vi "数据表比对.vi"(8 "error in (no error)":errorcluster, 9 "查询元素输入":string(combo), 10 "仪器日志参数":string, 11 "table输入":string(combo)) -> (0 "error out":errorcluster, 1 "columns输出":string[](array[string]), 2 "待发送第一条数据":string[](array[string]), 3 "待发送数据":string[][](table))   [LabVIEW 2016, in "数据传输系统-03.lvlib"]
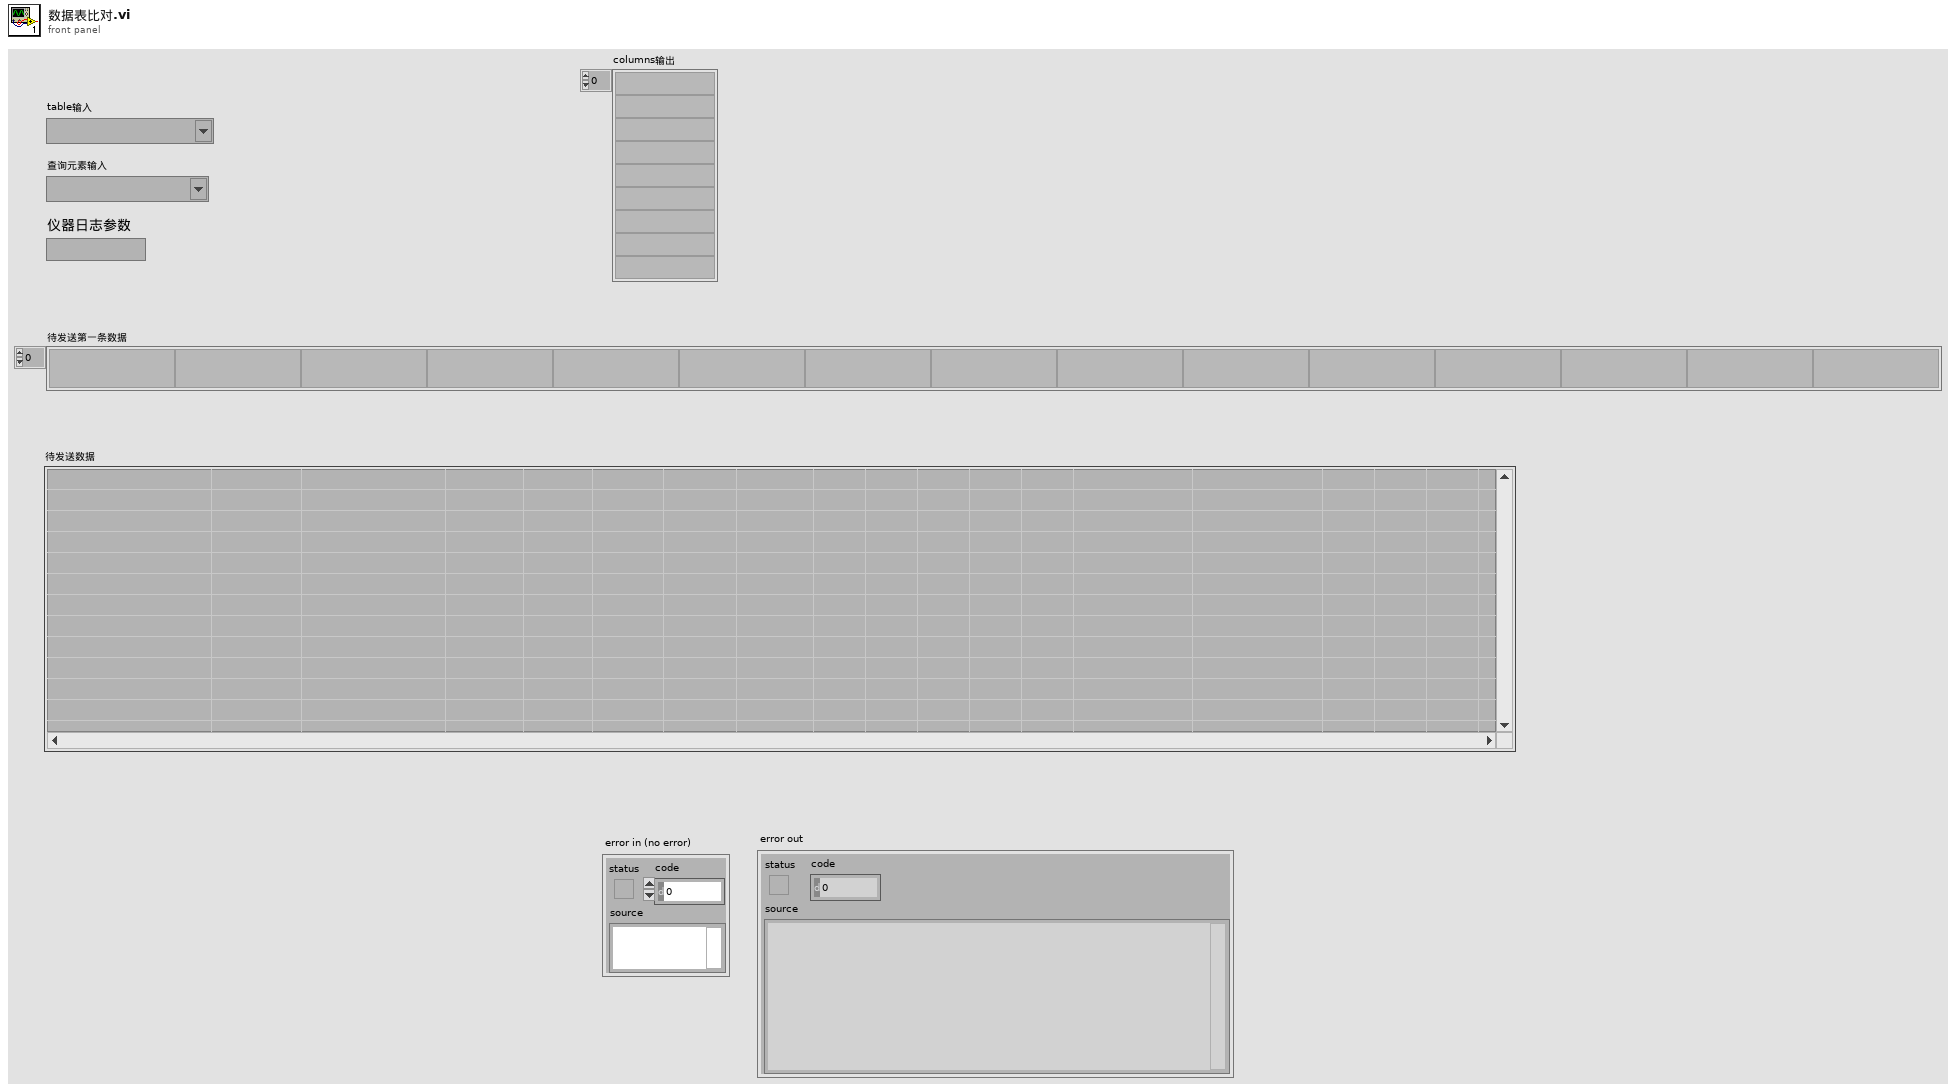
[diagram p1: front panel]
types:
  T1 = cluster{"氨氮仪器日志索引起始时间":string, "总磷仪器日志索引起始时间":string, "总氮仪器日志索引起始时间":string, "CODMn仪器日志索引起始时间":string, "CODCr仪器日志索引起始时间":string, "系统仪器日志索引起始时间":string, "氟化物仪器日志索引起始时间":string}
  T2 = cluster{"氨氮仪器参数索引起始时间":string, "总磷仪器参数索引起始时间":string, "总氮仪器参数索引起始时间":string, "CODMn仪器参数索引起始时间":string, "CODCr仪器参数索引起始时间":string, "DO仪器参数索引起始时间":string, "PH仪器参数索引起始时间":string, "比电导率仪器参数索引起始时间":string, "水温仪器参数索引起始时间":string, "浊度仪器参数索引起始时间":string, "叶绿素a仪器参数索引起始时间":string, "藻密度仪器参数索引起始时间":string, "ORP仪器参数索引起始时间":string, "氟化物仪器参数索引起始时间":string}
  T3 = cluster{"氨氮报警信息索引起始时间":string, "总磷报警信息索引起始时间":string, "总氮报警信息索引起始时间":string, "CODMn报警信息索引起始时间":string, "CODCr报警信息索引起始时间":string, "DO报警信息索引起始时间":string, "PH报警信息索引起始时间":string, "比电导率报警信息索引起始时间":string, "水温报警信息索引起始时间":string, "浊度报警信息索引起始时间":string, "叶绿素报警信息索引起始时间":string, "系统报警信息索引起始时间":string, "氟化物报警信息索引起始时间":string}
  T4 = cluster{"氨氮零点核查索引起始时间":string, "总磷零点核查索引起始时间":string, "总氮零点核查索引起始时间":string, "CODMn零点核查索引起始时间":string, "CODCr零点核查索引起始时间":string, "亚硝酸盐零点核查索引起始时间":string, "硫化物零点核查索引起始时间":string, "ORP零点核查索引起始时间":string, "氟化物零点核查索引起始时间":string}
  T5 = cluster{"氨氮标样核查索引起始时间":string, "总磷标样核查索引起始时间":string, "总氮标样核查索引起始时间":string, "CODMn标样核查索引起始时间":string, "CODCr标样核查索引起始时间":string, "DO标样核查索引起始时间":string, "PH标样核查索引起始时间":string, "比电导率标样核查索引起始时间":string, "水温标样核查索引起始时间":string, "浊度标样核查索引起始时间":string, "叶绿素a标样核查索引起始时间":string, "藻密度标样核查索引起始时间":string, "亚硝酸盐标样核查索引起始时间":string, "硫化物标样核查索引起始时间":string, "ORP标样核查索引起始时间":string, "氟化物标样核查索引起始时间":string}
  T6 = cluster{"氨氮跨度核查索引起始时间":string, "总磷跨度核查索引起始时间":string, "总氮跨度核查索引起始时间":string, "CODMn跨度核查索引起始时间":string, "CODCr跨度核查索引起始时间":string, "亚硝酸盐跨度核查索引起始时间":string, "硫化物跨度核查索引起始时间":string, "ORP跨度核查索引起始时间":string, "氟化物跨度核查索引起始时间":string}
  T7 = typedef "LVDateTimeRec.ctl" = cluster{"秒数的小数部分":dbl, "秒":i32, "分":i32, "时":i32, "日":i32, "月":i32, "年":i32, "天数（周）":i32, "天数（年）":i32, "DST":i32}
  T8 = cluster{"氨氮加标回收索引起始时间":string, "总磷加标回收索引起始时间":string, "总氮加标回收索引起始时间":string, "CODMn加标回收索引起始时间":string, "CODCr加标回收索引起始时间":string, "氟化物加标回收索引起始时间":string}
  T9 = cluster{"氨氮平行样索引起始时间":string, "总磷平行样索引起始时间":string, "总氮平行样索引起始时间":string, "CODMn平行样索引起始时间":string, "CODCr平行样索引起始时间":string, "氟化物平行样索引起始时间":string}
  T10 = cluster{"氨氮集成干预索引起始时间":string, "总磷集成干预索引起始时间":string, "总氮集成干预索引起始时间":string, "CODMn集成干预索引起始时间":string, "CODCr集成干预索引起始时间":string, "DO集成干预索引起始时间":string, "PH集成干预索引起始时间":string, "比电导率集成干预索引起始时间":string, "水温集成干预索引起始时间":string, "浊度集成干预索引起始时间":string, "叶绿素a集成干预索引起始时间":string, "藻密度集成干预索引起始时间":string, "亚硝酸盐集成干预索引起始时间":string, "硫化物集成干预索引起始时间":string, "ORP集成干预索引起始时间":string, "氟化物集成干预索引起始时间":string}
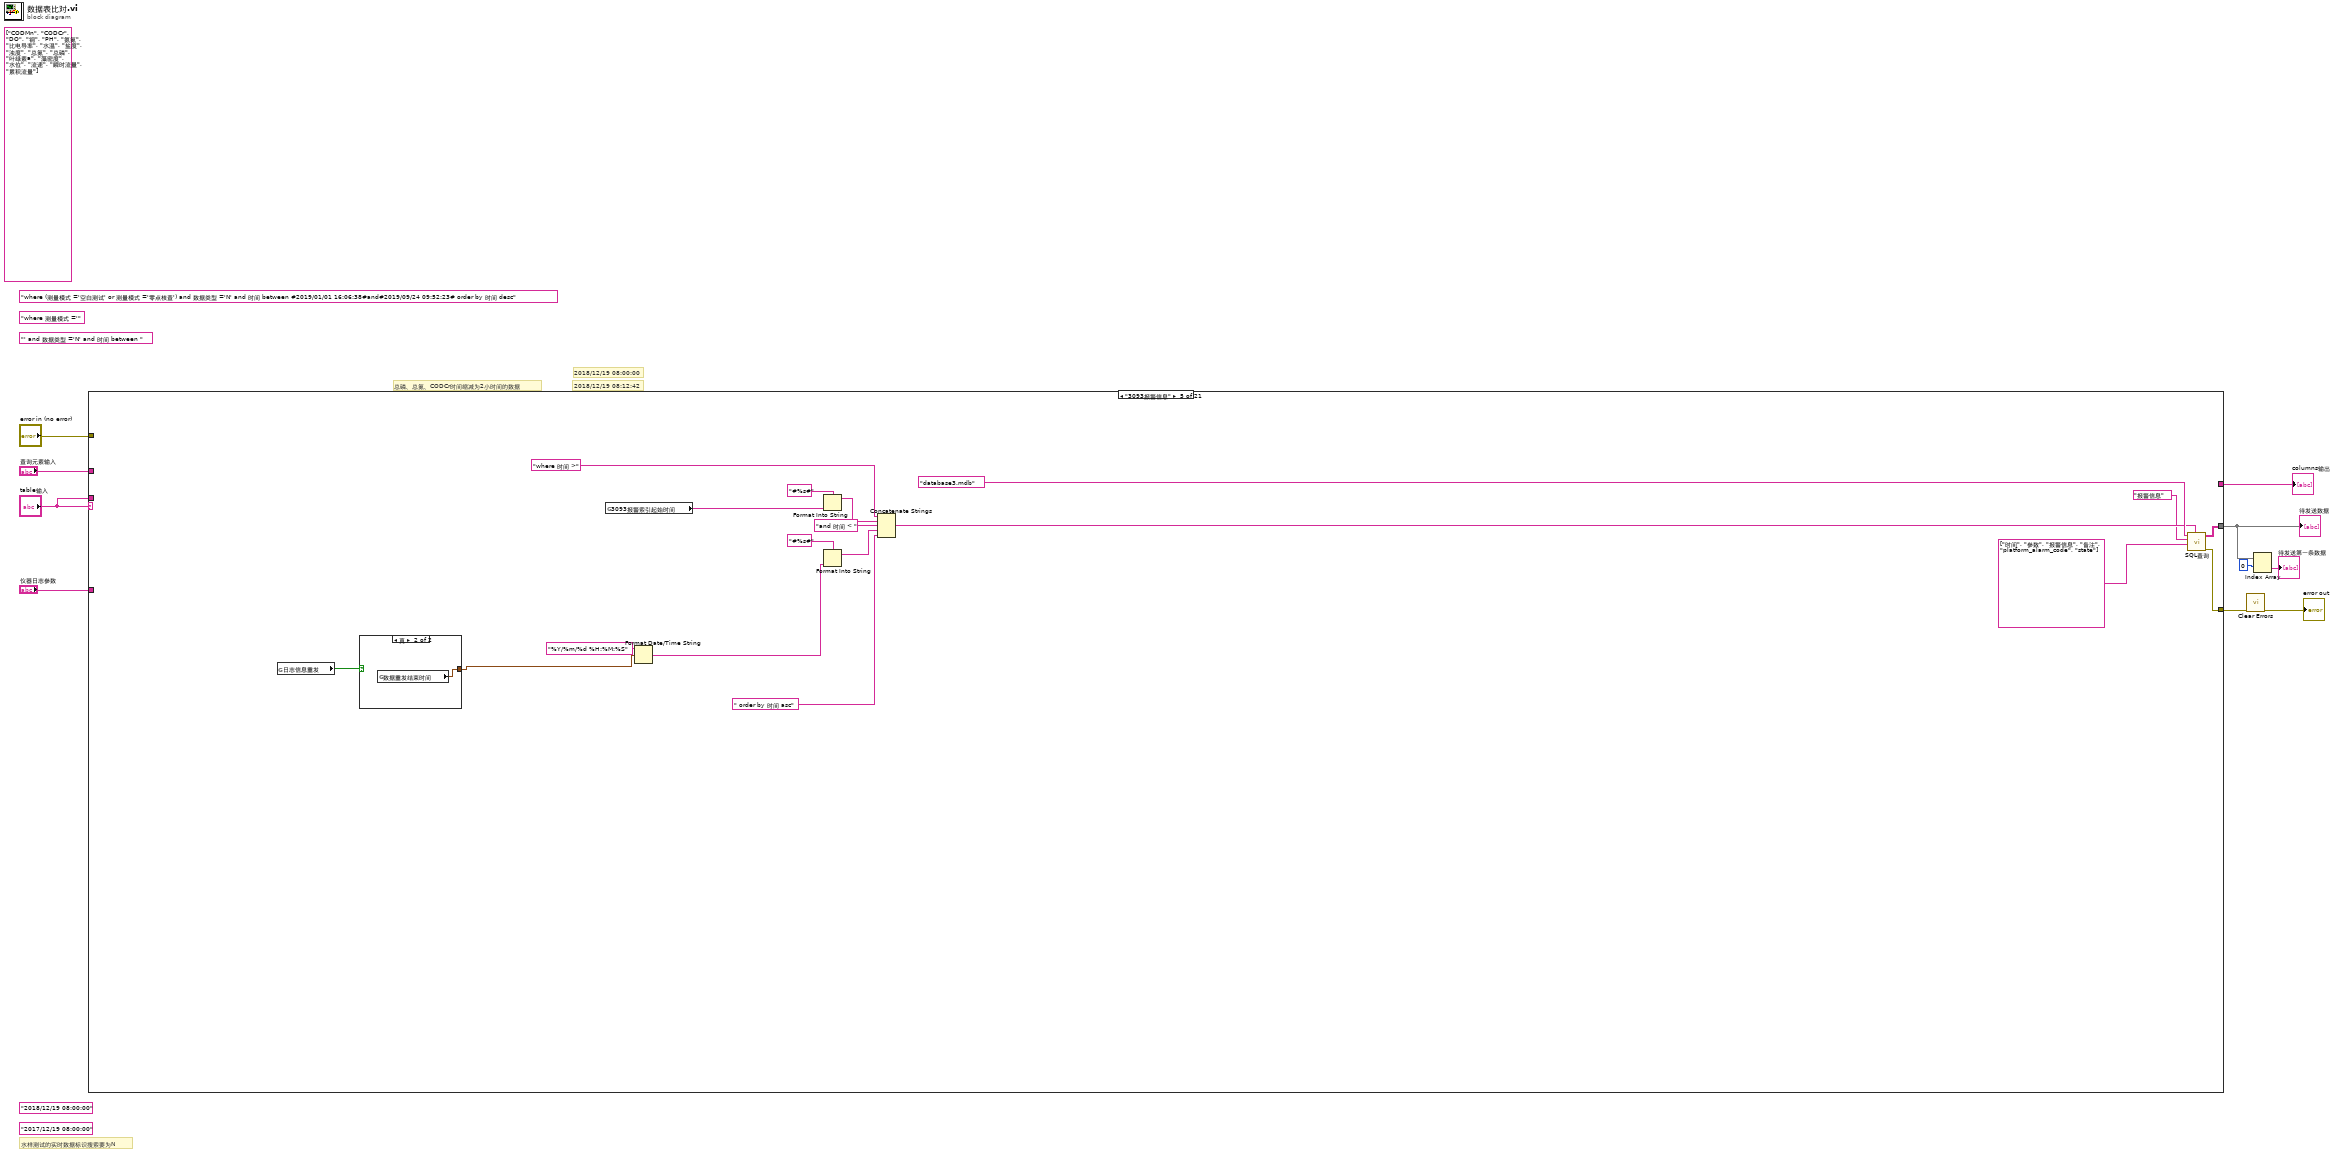
[diagram p0: block diagram]
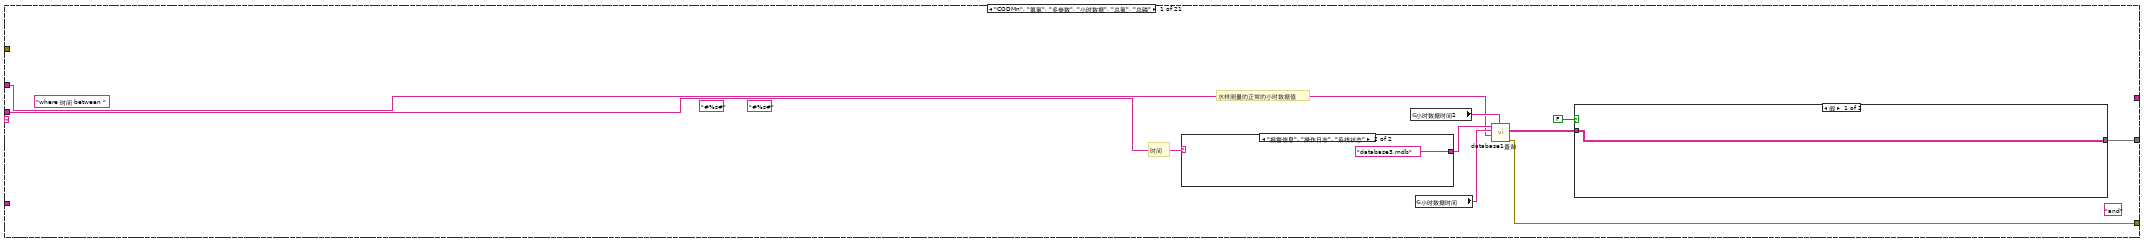
[diagram p2: hidden frame]
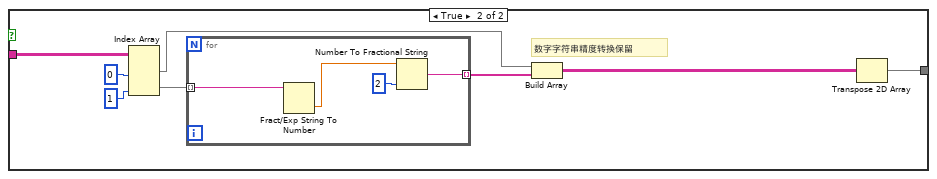
[diagram p3: hidden frame]
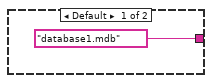
[diagram p4: hidden frame]
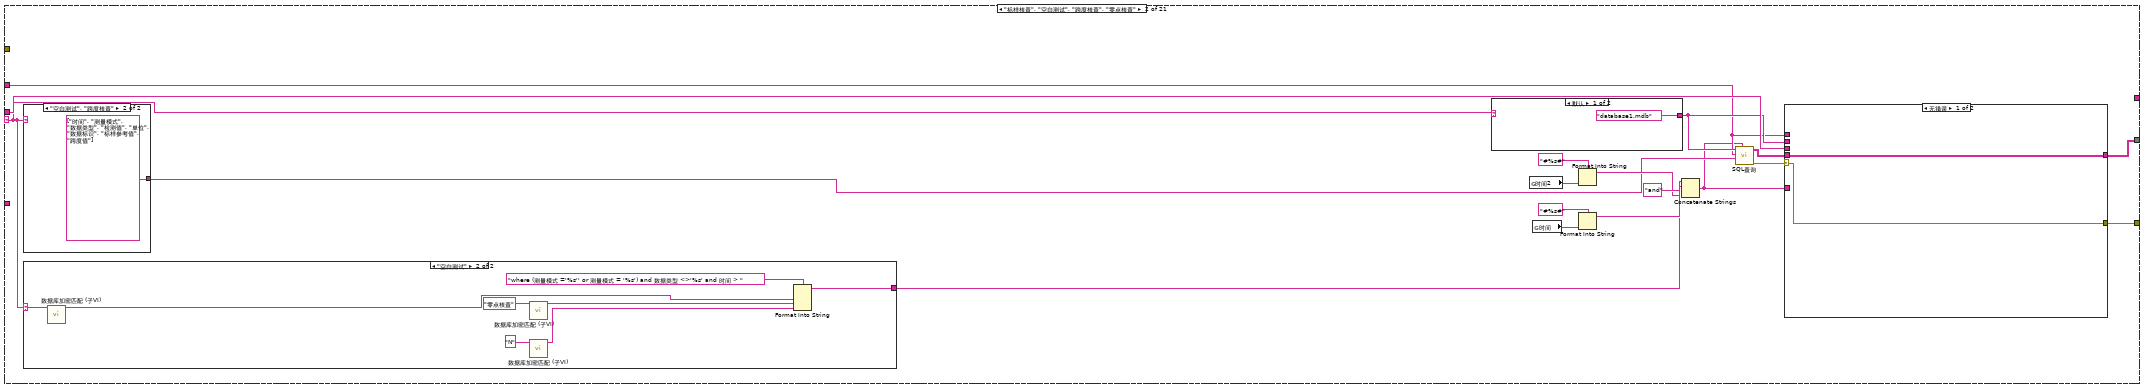
[diagram p5: hidden frame]
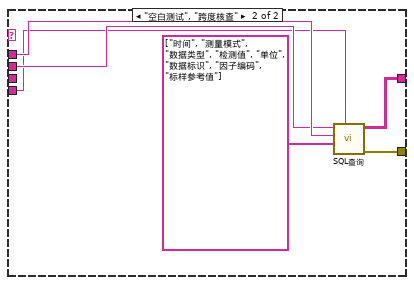
[diagram p7: hidden frame]
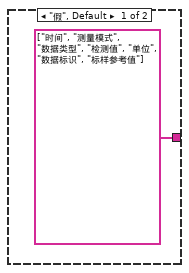
[diagram p8: hidden frame]
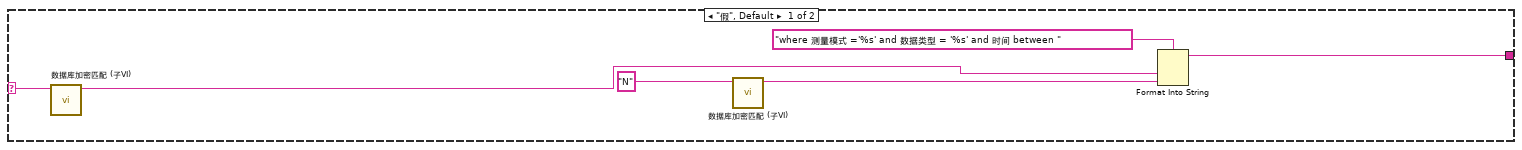
[diagram p9: hidden frame]
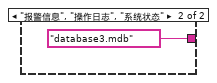
[diagram p10: hidden frame]
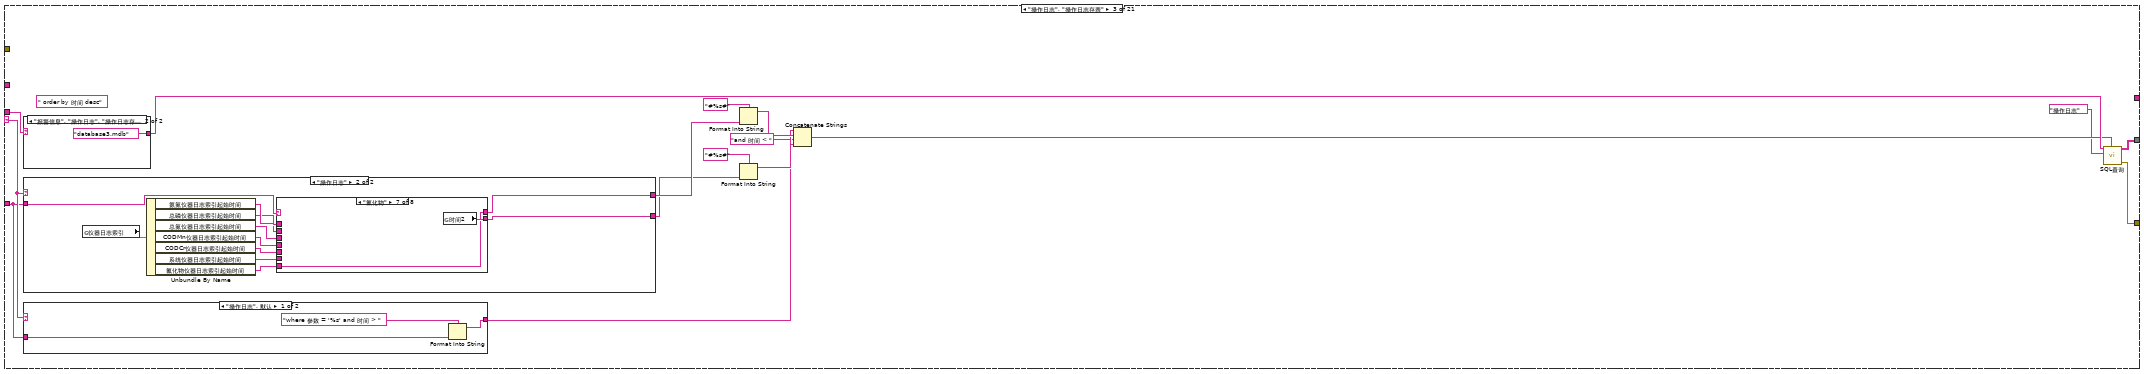
[diagram p11: hidden frame]
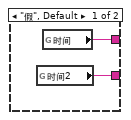
[diagram p12: hidden frame]
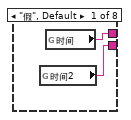
[diagram p13: hidden frame]
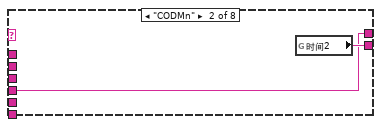
[diagram p14: hidden frame]
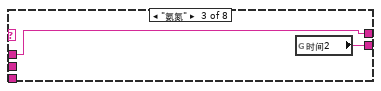
[diagram p15: hidden frame]
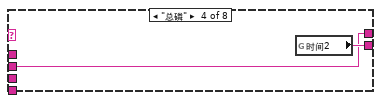
[diagram p16: hidden frame]
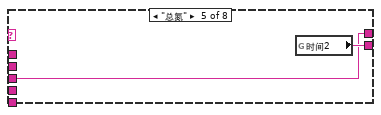
[diagram p17: hidden frame]
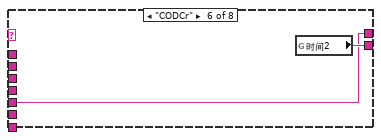
[diagram p18: hidden frame]
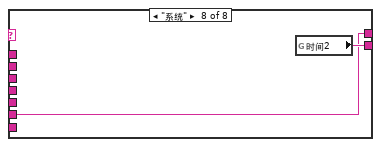
[diagram p19: hidden frame]
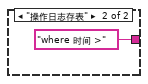
[diagram p20: hidden frame]
diagram:
  (unwired) "' and 数据类型 ='N' and 时间 between "
  (unwired) "where 测量模式 ='" ("condition")
  (unwired) "where (测量模式 ='空白测试' or 测量模式 ='零点核查') and 数据类型 ='N' and 时间 between #2019/01/01 16:06:38#and#2019/09/24 09:52:23# order by 时间 desc" ("condition")
  (unwired) string[] ["CODMn", "CODCr", "DO", "铜", "PH", "氨氮", "比电导率", "水温", "盐度", "浊度", "总氮", "总磷", "叶绿素a", "藻密度", "水位", "流速", "瞬时流量", "累积流量"] ("查询参数数组")
  (unwired) "2017/12/19 08:00:00"
  (unwired) "2018/12/19 08:00:00"
  # "水样测试的实时数据标识搜索要为N"
  # "2018/12/19 08:00:00"
  # "总磷、总氮、CODCr时间缩减为2小时间的数据"
  # "2018/12/19 08:12:42"
  n1 = case shown="\"3093报警信息\"" "table输入" {
    selector: "table输入" -> [_ w41 w91 _ _ _ _ _ _ w389 _ _ _ _ _ _ _ _ _ _ _]
    tunnel: "error in (no error)" -> [_ _ _ _ _ _ _ _ _ _ _ _ w500 _ _ _ _ _ _ _ _]
    tunnel: [w17 w35 w100 w153 w173 w192 w201 w260 w364 w403 w489 w497 w500 w501 w686 w731 w796 w865 w907 w950 w1001] -> w8
    tunnel: [w13 w36 w98 w151 w171 w190 w228 w262 w356 w401 w469 w496 w498 w503 w684 w734 w794 w868 w910 w953 w1003] -> w1
    tunnel: "table输入" -> [w19 w52 w102 _ _ _ w200 w263 _ w393 _ w493 _ _ _ _ _ _ _ _ _]
    tunnel: "查询元素输入" -> [w11 w39 _ _ _ _ _ _ _ _ _ _ _ w507 w671 w716 w782 w857 w899 w940 w997]
    tunnel: "仪器日志参数" -> [_ _ w88 _ _ w178 w195 w251 w335 w388 w468 _ _ _ _ _ _ _ _ _ _]
    tunnel: [_ _ _ _ _ _ _ _ _ _ _ w492 _ _ _ _ _ _ _ _ _] -> w2
    frame "CODMn", "氨氮", "多参数", "小时数据", "总氮", "总磷" {
      (unwired) "and" ("字符串")
      (unwired) "#%s#" ("初始字符串")
      (unwired) "#%s#" ("初始字符串")
      (unwired) "where 时间 between " ("condition")
      # "水样测量的正常的小时数据值"
      # "时间"
      n2 = case shown="\"报警信息\", \"操作日志\", \"系统状态\"" w19 {
        tunnel: ["database1.mdb" ("database") "database3.mdb" ("database")] -> w18
        frame Default {
        }
        frame "报警信息", "操作日志", "系统状态" {
        }
      }
      n3 = global read "全局 时间2.vi" "小时数据时间2"() -> (w15:string)
      n4 = global read "全局 水样时间.vi" "小时数据时间"() -> (w16:string)
      n5 = call "database1查询.vi"("时间2"=w15, "table"=w11, "时间1"=w16, "database"=w18) -> ("error out"=w17:errorcluster, "data"=w14:string[][])  [unwired: 4 in, 1 out]
      n6 = case shown="假" FALSE {
        tunnel: w14 -> [w20 w28]
        tunnel: [w20 w21] -> w13
        frame False {
        }
        frame True {
          # "数字字符串精度转换保留"
          n7 = Index Array(array=w28, index (col) #1=0 ("禁用的索引 (列)"), index (col) #2=1 ("索引 (列)")) -> (element #1=w24:string[], element #2=w25:string[])  [unwired: 2 in]
          n8 = for {
            tunnel: w25 -> [w30] mode=indexing
            tunnel: [w29] -> w23 mode=indexing
            n9 = Fract/Exp String To Number(string=w30) -> (number=w31:dbl)  [unwired: 3 in, 1 out]
            n10 = Number To Fractional String(number=w31, precision (6)=i16 2 ("精度(6)")) -> (F-format string=w29:string)  [unwired: 2 in]
          }
          n11 = Build Array(w24, w23) -> (w22:string[][])
          n12 = Transpose 2D Array(2D array=w22) -> (transposed array=w21:string[][])
        }
      }
    }
    frame "标样核查", "空白测试", "跨度核查", "零点核查" {
      n13 = case shown="\"空白测试\", \"跨度核查\"" w41 {
        tunnel: [string[] ["时间", "测量模式", "数据类型", "检测值", "单位", "数据标识", "标样参考值"] ("columns") string[] ["时间", "测量模式", "数据类型", "检测值", "单位", "数据标识", "标样参考值", "跨度值"] ("columns")] -> w43
        frame "假", Default {
        }
        frame "空白测试", "跨度核查" {
        }
      }
      n14 = case shown="\"空白测试\"" w41 {
        selector: w41 -> [w74 w81]
        tunnel: [w75 w83] -> w44
        frame "假", Default {
          n15 = call "数据库加密匹配 (子VI).vi"("输入参数"=w74) -> ("Encoded String"=w73:string)  [unwired: 10 in]
          n16 = call "数据库加密匹配 (子VI).vi"("输入参数"="N" ("字符串")) -> ("Encoded String"=w71:string)  [unwired: 10 in]
          n17 = Format Into String(format string="where 测量模式 ='%s' and 数据类型 = '%s' and 时间 between " ("格式字符串"), w73, w71) -> (resulting string=w75:string)  [unwired: 2 in, 1 out]
        }
        frame "空白测试" {
          n18 = call "数据库加密匹配 (子VI).vi"("输入参数"=w81) -> ("Encoded String"=w82:string)  [unwired: 10 in]
          n19 = call "数据库加密匹配 (子VI).vi"("输入参数"="零点核查") -> ("Encoded String"=w79:string)  [unwired: 10 in]
          n20 = call "数据库加密匹配 (子VI).vi"("输入参数"="N") -> ("Encoded String"=w77:string)  [unwired: 10 in]
          n21 = Format Into String(format string="where (测量模式 ='%s'' or 测量模式 = '%s') and 数据类型 <>'%s' and 时间 > " ("格式字符串"), w82, w79, w77) -> (resulting string=w83:string)  [unwired: 2 in, 1 out]
        }
      }
      n22 = case shown="默认" w52 {
        tunnel: ["database1.mdb" ("database") "database3.mdb" ("database")] -> w40
        frame Default {
        }
        frame "报警信息", "操作日志", "系统状态" {
        }
      }
      n23 = global read "全局 时间2.vi" "时间2"() -> (w45:string)
      n24 = global read "全局 水样时间.vi" "时间"() -> (w46:string)
      n25 = Format Into String(format string="#%s#" ("初始字符串"), w45) -> (resulting string=w47:string)  [unwired: 2 in, 1 out]
      n26 = Format Into String(format string="#%s#" ("初始字符串"), w46) -> (resulting string=w51:string)  [unwired: 2 in, 1 out]
      n27 = Concatenate Strings(w44, w51, "and" ("字符串"), w47) -> (w38:string)
      n28 = call "SQL查询.vi"("condition"=w38, "columns"=w43, "table输入"=w39, "database"=w40) -> ("error out"=w42:errorcluster, "data"=w37:string[][])  [unwired: 4 in, 2 out]
      n29 = case shown="无错误" w42 {
        selector: w42 -> [w53 _]
        tunnel: w41 -> [_ w61]
        tunnel: w39 -> [_ w60]
        tunnel: w40 -> [_ w59]
        tunnel: w38 -> [_ w58]
        tunnel: w37 -> [w54 w56]
        tunnel: [w54 w57] -> w36
        tunnel: [w53 w55] -> w35
        frame No Error {
        }
        frame Error {
          # "兼容旧数据库没有跨度值版本"
          n30 = case shown="\"假\", 默认" w61 {
            tunnel: w60 -> [_ w67]
            tunnel: w59 -> [_ w66]
            tunnel: w58 -> [_ w65]
            tunnel: [w62 w64] -> w57
            tunnel: w56 -> [w62 _]
            tunnel: [_ w63] -> w55
            frame "假", Default {
            }
            frame "空白测试", "跨度核查" {
              n31 = call "SQL查询.vi"("condition"=w65, "columns"=string[] ["时间", "测量模式", "数据类型", "检测值", "单位", "数据标识", "因子编码", "标样参考值"], "table输入"=w67, "database"=w66) -> ("error out"=w63:errorcluster, "data"=w64:string[][])  [unwired: 4 in, 2 out]
            }
          }
        }
      }
    }
    frame "操作日志", "操作日志存表" {
      (unwired) " order by 时间 desc" ("字符串")
      n32 = case shown="\"报警信息\", \"操作日志\", \"操作日志存表\", \"系统状态\"" w102 {
        tunnel: ["database1.mdb" ("database") "database3.mdb" ("database")] -> w101
        frame Default {
        }
        frame "报警信息", "操作日志", "操作日志存表", "系统状态" {
        }
      }
      n33 = case shown="\"操作日志\"" w91 {
        tunnel: [w104 w114] -> w90
        tunnel: [w103 w106] -> w89
        tunnel: w88 -> [_ w115]
        frame "假", Default {
          n34 = global read "全局 时间2.vi" "时间2"() -> (w103:string)
          n35 = global read "全局 水样时间.vi" "时间"() -> (w104:string)
        }
        frame "操作日志" {
          n36 = global read "全局 时间2.vi" "仪器日志索引"() -> (w113:T1)
          n37 = Unbundle By Name(w113) -> ("氨氮仪器日志索引起始时间"=w112:string, "总磷仪器日志索引起始时间"=w111:string, "总氮仪器日志索引起始时间"=w110:string, "CODMn仪器日志索引起始时间"=w109:string, "CODCr仪器日志索引起始时间"=w108:string, "系统仪器日志索引起始时间"=w107:string, "氟化物仪器日志索引起始时间"=w105:string)
          n38 = case shown="\"氟化物\"" w115 {
            tunnel: [w116 w119 w121 w123 w125 w127 w129 w131] -> w106
            tunnel: [w117 w118 w120 w122 w124 w126 w128 w130] -> w114
            tunnel: w112 -> [_ _ w120 _ _ _ _ _]
            tunnel: w111 -> [_ _ _ w122 _ _ _ _]
            tunnel: w110 -> [_ _ _ _ w124 _ _ _]
            tunnel: w109 -> [_ w118 _ _ _ _ _ _]
            tunnel: w108 -> [_ _ _ _ _ w126 _ _]
            tunnel: w107 -> [_ _ _ _ _ _ _ w130]
            tunnel: w105 -> [_ _ _ _ _ _ w128 _]
            frame "假", Default {
              n39 = global read "全局 时间2.vi" "时间2"() -> (w116:string)
              n40 = global read "全局 水样时间.vi" "时间"() -> (w117:string)
            }
            frame "CODMn" {
              n41 = global read "全局 时间2.vi" "时间2"() -> (w119:string)
            }
            frame "氨氮" {
              n42 = global read "全局 时间2.vi" "时间2"() -> (w121:string)
            }
            frame "总磷" {
              n43 = global read "全局 时间2.vi" "时间2"() -> (w123:string)
            }
            frame "总氮" {
              n44 = global read "全局 时间2.vi" "时间2"() -> (w125:string)
            }
            frame "CODCr" {
              n45 = global read "全局 时间2.vi" "时间2"() -> (w127:string)
            }
            frame "氟化物" {
              n46 = global read "全局 时间2.vi" "时间2"() -> (w129:string)
            }
            frame "系统" {
              n47 = global read "全局 时间2.vi" "时间2"() -> (w131:string)
            }
          }
        }
      }
      n48 = case shown="\"操作日志\", 默认" w91 {
        tunnel: [w133 "where 时间 >" ("condition")] -> w93
        tunnel: w88 -> [w132 _]
        frame "操作日志", Default {
          n49 = Format Into String(format string="where 参数 = '%s' and 时间 > " ("condition"), w132) -> (resulting string=w133:string)  [unwired: 2 in, 1 out]
        }
        frame "操作日志存表" {
        }
      }
      n50 = Format Into String(format string="#%s#" ("初始字符串"), w90) -> (resulting string=w97:string)  [unwired: 2 in, 1 out]
      n51 = Format Into String(format string="#%s#" ("初始字符串"), w89) -> (resulting string=w94:string)  [unwired: 2 in, 1 out]
      n52 = Concatenate Strings(w93, w97, "and 时间 < " ("字符串"), w94) -> (w99:string)
      n53 = call "SQL查询.vi"("condition"=w99, "table输入"="操作日志", "database"=w101) -> ("error out"=w100:errorcluster, "data"=w98:string[][])  [unwired: 5 in, 2 out]
    }
    frame "3092日志信息" {
      n54 = global read "断电保存全局.vi" "日志信息重发"() -> (w138:bool)
      n55 = case shown="真" w138 {
        tunnel: [w155 w156] -> w141
        frame False {
          n56 = Get Date/Time In Seconds() -> (seconds since 1Jan1904=w155:timestamp)
        }
        frame True {
          n57 = global read "断电保存全局.vi" "数据重发结束时间"() -> (w156:timestamp)
        }
      }
      n58 = global read "全局 时间2.vi" "3092日志索引起始时间"() -> (w143:string)
      n59 = Format Date/Time String(time format string (%c)="%Y/%m/%d %H:%M:%S" ("时间格式字符串(%c)"), seconds (now)=w141) -> (date/time string=w140:string)  [unwired: 1 in]
      n60 = Format Into String(format string="#%s#" ("初始字符串"), w143) -> (resulting string=w150:string)  [unwired: 2 in, 1 out]
      n61 = Format Into String(format string="#%s#" ("初始字符串"), w140) -> (resulting string=w147:string)  [unwired: 2 in, 1 out]
      n62 = Concatenate Strings("where 时间 >" ("condition"), w150, "and 时间 < " ("字符串"), w147, " order by 时间 asc" ("字符串")) -> (w152:string)
      n63 = call "SQL查询.vi"("condition"=w152, "table输入"="操作日志", "database"="database3.mdb") -> ("error out"=w153:errorcluster, "data"=w151:string[][])  [unwired: 5 in, 2 out]
    }
    frame "3093报警信息" {
      n64 = global read "断电保存全局.vi" "日志信息重发"() -> (w158:bool)
      n65 = case shown="真" w158 {
        tunnel: [w175 w176] -> w157
        frame False {
          n66 = Get Date/Time In Seconds() -> (seconds since 1Jan1904=w175:timestamp)
        }
        frame True {
          n67 = global read "断电保存全局.vi" "数据重发结束时间"() -> (w176:timestamp)
        }
      }
      n68 = global read "全局 时间2.vi" "3093报警索引起始时间"() -> (w163:string)
      n69 = Format Date/Time String(time format string (%c)="%Y/%m/%d %H:%M:%S" ("时间格式字符串(%c)"), seconds (now)=w157) -> (date/time string=w161:string)  [unwired: 1 in]
      n70 = Format Into String(format string="#%s#" ("初始字符串"), w163) -> (resulting string=w170:string)  [unwired: 2 in, 1 out]
      n71 = Format Into String(format string="#%s#" ("初始字符串"), w161) -> (resulting string=w167:string)  [unwired: 2 in, 1 out]
      n72 = Concatenate Strings("where 时间 >" ("condition"), w170, "and 时间 < " ("字符串"), w167, " order by 时间 asc" ("字符串")) -> (w172:string)
      n73 = call "SQL查询.vi"("condition"=w172, "columns"=string[] ["时间", "参数", "报警信息", "备注", "platform_alarm_code", "state"], "table输入"="报警信息", "database"="database3.mdb") -> ("error out"=w173:errorcluster, "data"=w171:string[][])  [unwired: 4 in, 2 out]
    }
    frame "提取操作日志" {
      n74 = call "数据库加密匹配 (子VI).vi"("输入参数"=w178) -> ("Encoded String"=w177:string)  [unwired: 10 in]
      n75 = global read "全局 时间2.vi" "时间2"() -> (w181:string)
      n76 = global read "全局 水样时间.vi" "时间"() -> (w182:string)
      n77 = Format Into String(format string="where 参数 = '%s' and 时间 between" ("condition"), w177) -> (resulting string=w184:string)  [unwired: 2 in, 1 out]
      n78 = Format Into String(format string="#%s#" ("初始字符串"), w182) -> (resulting string=w189:string)  [unwired: 2 in, 1 out]
      n79 = Format Into String(format string="#%s#" ("初始字符串"), w181) -> (resulting string=w185:string)  [unwired: 2 in, 1 out]
      n80 = Concatenate Strings(w184, w189, "and" ("字符串"), w185) -> (w191:string)
      n81 = call "SQL查询.vi"("condition"=w191, "table输入"="操作日志", "database"="database3.mdb") -> ("error out"=w192:errorcluster, "data"=w190:string[][])  [unwired: 5 in, 2 out]
    }
    frame "3090仪器参数" {
      (unwired) string[] ["时间", "参数", "测量量程", "测量精度", "测量间隔", "消解温度", "消解时长", "空白校准时间", "曲线截距", "曲线斜率", "测量检出限", "测量信号值", "线性相关系数", "二次多项式系数", "标样校准时间", "稀释倍数", "三项式系数", "空白标定系数", "量程系数", "F0/ORPA", "F1/ORPB", "F2/ORPK", "F3", "F4", "F5", "F6", "F7", "X0/滴定数", "量程"] ("columns输出")
      n82 = case shown="\"3090仪器参数\"" w200 {
        tunnel: [w231 w232] -> w216
        frame "3090仪器参数" {
          n83 = global read "全局 时间2.vi" "3090仪器参数索引"() -> (w231:T2)
        }
        frame "仪器参数", Default {
          n84 = global read "全局 时间2.vi" "仪器参数索引"() -> (w232:T2)
        }
      }
      n85 = call "数据库加密匹配 (子VI).vi"("输入参数"=w195) -> ("Encoded String"=w194:string)  [unwired: 10 in]
      n86 = global read "断电保存全局.vi" "数据发送延时时间/s"() -> (w197:i32)
      n87 = Unbundle By Name(w216) -> ("氨氮仪器参数索引起始时间"=w215:string, "总磷仪器参数索引起始时间"=w214:string, "总氮仪器参数索引起始时间"=w213:string, "CODMn仪器参数索引起始时间"=w212:string, "CODCr仪器参数索引起始时间"=w211:string, "DO仪器参数索引起始时间"=w209:string, "PH仪器参数索引起始时间"=w208:string, "比电导率仪器参数索引起始时间"=w207:string, "水温仪器参数索引起始时间"=w206:string, "浊度仪器参数索引起始时间"=w205:string, "叶绿素a仪器参数索引起始时间"=w204:string, "藻密度仪器参数索引起始时间"=w203:string, "ORP仪器参数索引起始时间"=w202:string, "氟化物仪器参数索引起始时间"=w193:string)
      n88 = Format Into String(format string="where 参数 = '%s' and 时间 > " ("condition"), w194) -> (resulting string=w223:string)  [unwired: 2 in, 1 out]
      n89 = Get Date/Time In Seconds() -> (seconds since 1Jan1904=w198:timestamp)
      n90 = case shown="\"氟化物\"" w195 {
        tunnel: w215 -> [_ _ w235 _ _ _ _ _ _ _ _ _ _ _ _]
        tunnel: w214 -> [_ _ _ w236 _ _ _ _ _ _ _ _ _ _ _]
        tunnel: w213 -> [_ _ _ _ w237 _ _ _ _ _ _ _ _ _ _]
        tunnel: w212 -> [w233 w234 _ _ _ _ _ _ _ _ _ _ _ _ _]
        tunnel: w211 -> [_ _ _ _ _ w238 _ _ _ _ _ _ _ _ _]
        tunnel: [w233 w234 w235 w236 w237 w238 w239 w240 w241 w242 w243 w244 w245 w246 w247] -> w210
        tunnel: w209 -> [_ _ _ _ _ _ w239 _ _ _ _ _ _ _ _]
        tunnel: w208 -> [_ _ _ _ _ _ _ w240 _ _ _ _ _ _ _]
        tunnel: w207 -> [_ _ _ _ _ _ _ _ w241 _ _ _ _ _ _]
        tunnel: w206 -> [_ _ _ _ _ _ _ _ _ w242 _ _ _ _ _]
        tunnel: w205 -> [_ _ _ _ _ _ _ _ _ _ w243 _ _ _ _]
        tunnel: w204 -> [_ _ _ _ _ _ _ _ _ _ _ w244 _ _ _]
        tunnel: w203 -> [_ _ _ _ _ _ _ _ _ _ _ _ w245 _ _]
        tunnel: w202 -> [_ _ _ _ _ _ _ _ _ _ _ _ _ w246 _]
        tunnel: w193 -> [_ _ _ _ _ _ _ _ _ _ _ _ _ _ w247]
        frame "假", Default {
        }
        frame "CODMn" {
        }
        frame "氨氮" {
        }
        frame "总磷" {
        }
        frame "总氮" {
        }
        frame "CODCr" {
        }
        frame "溶解氧" {
        }
        frame "PH" {
        }
        frame "电导率" {
        }
        frame "水温" {
        }
        frame "浊度" {
        }
        frame "叶绿素" {
        }
        frame "藻密度" {
        }
        frame "ORP" {
        }
        frame "氟化物" {
        }
      }
      n91 = Subtract(x=w198, y=w197) -> (x-y=w196:timestamp)
      n92 = Format Date/Time String(time format string (%c)="%Y/%m/%d %H:%M:%S" ("时间格式字符串(%c)"), seconds (now)=w196) -> (date/time string=w219:string)  [unwired: 1 in]
      n93 = Search and Replace String(input string=w219, search string="." ("搜索字符串")) -> (result string=w217:string)  [unwired: 6 in, 3 out]
      n94 = Format Into String(format string="#%s#" ("初始字符串"), w217) -> (resulting string=w224:string)  [unwired: 2 in, 1 out]
      n95 = Format Into String(format string="#%s#" ("初始字符串"), w210) -> (resulting string=w227:string)  [unwired: 2 in, 1 out]
      n96 = Concatenate Strings(w223, w227, "and 时间 < " ("字符串"), w224, " order by 时间 asc" ("字符串")) -> (w229:string)
      n97 = call "SQL查询.vi"("condition"=w229, "table输入"=w200, "database"="database3.mdb") -> ("error out"=w201:errorcluster, "data"=w228:string[][])  [unwired: 5 in, 2 out]
    }
    frame "仪器参数" {
      n98 = case shown="\"仪器参数\", 默认" w263 {
        tunnel: [w318 w319] -> w280
        frame "3090仪器参数" {
          n99 = global read "全局 时间2.vi" "3090仪器参数索引"() -> (w318:T2)
        }
        frame "仪器参数", Default {
          n100 = global read "全局 时间2.vi" "仪器参数索引"() -> (w319:T2)
        }
      }
      n101 = Unbundle By Name(w280) -> ("氨氮仪器参数索引起始时间"=w279:string, "总磷仪器参数索引起始时间"=w278:string, "总氮仪器参数索引起始时间"=w277:string, "CODMn仪器参数索引起始时间"=w276:string, "CODCr仪器参数索引起始时间"=w275:string, "DO仪器参数索引起始时间"=w274:string, "PH仪器参数索引起始时间"=w273:string, "比电导率仪器参数索引起始时间"=w272:string, "水温仪器参数索引起始时间"=w271:string, "浊度仪器参数索引起始时间"=w270:string, "叶绿素a仪器参数索引起始时间"=w269:string, "藻密度仪器参数索引起始时间"=w268:string, "ORP仪器参数索引起始时间"=w267:string, "氟化物仪器参数索引起始时间"=w248:string)
      n102 = case shown="\"氟化物\"" w251 {
        tunnel: w279 -> [_ _ w322 _ _ _ _ _ _ _ _ _ _ _ _]
        tunnel: w278 -> [_ _ _ w323 _ _ _ _ _ _ _ _ _ _ _]
        tunnel: w277 -> [_ _ _ _ w324 _ _ _ _ _ _ _ _ _ _]
        tunnel: w276 -> [w320 w321 _ _ _ _ _ _ _ _ _ _ _ _ _]
        tunnel: w275 -> [_ _ _ _ _ w325 _ _ _ _ _ _ _ _ _]
        tunnel: [w320 w321 w322 w323 w324 w325 w326 w327 w328 w329 w330 w331 w332 w333 w334] -> w265
        tunnel: w274 -> [_ _ _ _ _ _ w326 _ _ _ _ _ _ _ _]
        tunnel: w273 -> [_ _ _ _ _ _ _ w327 _ _ _ _ _ _ _]
        tunnel: w272 -> [_ _ _ _ _ _ _ _ w328 _ _ _ _ _ _]
        tunnel: w271 -> [_ _ _ _ _ _ _ _ _ w329 _ _ _ _ _]
        tunnel: w270 -> [_ _ _ _ _ _ _ _ _ _ w330 _ _ _ _]
        tunnel: w269 -> [_ _ _ _ _ _ _ _ _ _ _ w331 _ _ _]
        tunnel: w268 -> [_ _ _ _ _ _ _ _ _ _ _ _ w332 _ _]
        tunnel: w267 -> [_ _ _ _ _ _ _ _ _ _ _ _ _ w333 _]
        tunnel: w248 -> [_ _ _ _ _ _ _ _ _ _ _ _ _ _ w334]
        frame "假", Default {
        }
        frame "CODMn" {
        }
        frame "氨氮" {
        }
        frame "总磷" {
        }
        frame "总氮" {
        }
        frame "CODCr" {
        }
        frame "溶解氧" {
        }
        frame "PH" {
        }
        frame "电导率" {
        }
        frame "水温" {
        }
        frame "浊度" {
        }
        frame "叶绿素" {
        }
        frame "藻密度" {
        }
        frame "ORP" {
        }
        frame "氟化物" {
        }
      }
      n103 = Format Into String(format string="#%s#" ("初始字符串"), w265) -> (resulting string=w288:string)  [unwired: 2 in, 1 out]
      n104 = global read "断电保存全局.vi" "日志信息重发"() -> (w250:bool)
      n105 = case shown="假" w250 {
        tunnel: [w291 w294] -> w249
        frame False {
          n106 = global read "断电保存全局.vi" "数据发送延时时间/s"() -> (w292:i32)
          n107 = Get Date/Time In Seconds() -> (seconds since 1Jan1904=w293:timestamp)
          n108 = Subtract(x=w293, y=w292) -> (x-y=w291:timestamp)
        }
        frame True {
          n109 = global read "断电保存全局.vi" "数据重发结束时间"() -> (w294:timestamp)
        }
      }
      n110 = global read "断电保存全局.vi" "应用环境"() -> (w253:enum16{"STD", "GB212"})
      n111 = call "数据库加密匹配 (子VI).vi"("输入参数"="N") -> ("Encoded String"=w254:string)  [unwired: 10 in]
      n112 = case shown="\"STD\"" w253 {
        tunnel: [w296 string[] ["时间", "数据类型", "测量量程", "测量精度", "测量间隔", "消解温度", "消解时长", "空白校准时间", "曲线截距", "曲线斜率", "测量检出限", "测量信号值", "线性相关系数", "二次多项式系数", "标样校准时间"] ("columns输出")] -> w266
        tunnel: w251 -> [w295 _]
        frame "STD" {
          n113 = case shown="\"CODMn\"" w295 {
            tunnel: [string[] ["时间", "数据类型", "测量量程", "测量精度", "测量间隔", "消解温度", "消解时长", "空白校准时间", "曲线截距", "曲线斜率", "测量检出限", "测量信号值", "线性相关系数", "二次多项式系数", "标样校准时间", "量程"] ("columns输出") string[] ["时间", "数据类型", "测量量程", "测量精度", "测量间隔", "消解温度", "消解时长", "空白校准时间", "曲线截距", "曲线斜率", "测量检出限", "测量信号值", "线性相关系数", "二次多项式系数", "标样校准时间", "量程标识"] ("columns输出")] -> w296
            frame "CODMn" {
            }
            frame "", Default {
            }
          }
        }
        frame "GB212", Default {
        }
      }
      n114 = Format Date/Time String(time format string (%c)="%Y/%m/%d %H:%M:%S" ("时间格式字符串(%c)"), seconds (now)=w249) -> (date/time string=w282:string)  [unwired: 1 in]
      n115 = Search and Replace String(input string=w282, search string="." ("搜索字符串")) -> (result string=w264:string)  [unwired: 6 in, 3 out]
      n116 = Format Into String(format string="where 数据类型 = '%s' and 时间 > " ("condition"), w254) -> (resulting string=w256:string)  [unwired: 2 in, 1 out]
      n117 = Format Into String(format string="#%s#" ("初始字符串"), w264) -> (resulting string=w285:string)  [unwired: 2 in, 1 out]
      n118 = Concatenate Strings(w256, w288, "and 时间 < " ("字符串"), w285, " order by 时间 asc" ("字符串")) -> (w289:string)
      n119 = call "SQL查询.vi"("condition"=w289, "columns"=w266, "table输入"=w251, "database"="database1.mdb") -> ("error out"=w259:errorcluster, "data"=w261:string[][])  [unwired: 4 in, 2 out]
      n120 = Empty Array?(array=w261) -> ()  [unwired: 1 out]
      n121 = case shown="假" FALSE {
        tunnel: w251 -> [_ w315]
        tunnel: w265 -> [_ w311]
        tunnel: w264 -> [_ w307]
        tunnel: w263 -> [_ w304]
        tunnel: [w301 w303] -> w262
        tunnel: w261 -> [w301 _]
        tunnel: [w300 w302] -> w260
        tunnel: w259 -> [w300 _]
        frame False {
        }
        frame True {
          n122 = Format Into String(format string="#%s#" ("初始字符串"), w307) -> (resulting string=w306:string)  [unwired: 2 in, 1 out]
          n123 = Format Into String(format string="#%s#" ("初始字符串"), w311) -> (resulting string=w310:string)  [unwired: 2 in, 1 out]
          n124 = Format Into String(format string="where 参数 = '%s' and 时间 between" ("condition"), w315) -> (resulting string=w313:string)  [unwired: 2 in, 1 out]
          n125 = Concatenate Strings(w313, w310, "and" ("字符串"), w306, " order by 时间 asc" ("字符串")) -> (w314:string)
          n126 = call "SQL查询.vi"("condition"=w314, "table输入"=w304, "database"="database3.mdb") -> ("error out"=w302:errorcluster, "data"=w303:string[][])  [unwired: 5 in, 2 out]
        }
      }
    }
    frame "提取仪器参数" {
      w358 = 0 ("索引 (行)")
      n127 = call "数据库加密匹配 (子VI).vi"("输入参数"=w335) -> ("Encoded String"=w338:string)  [unwired: 10 in]
      n128 = global read "断电保存全局.vi" "应用环境"() -> (w336:enum16{"STD", "GB212"})
      n129 = case shown="\"STD\"" w336 {
        tunnel: [w366 string[] ["时间", "数据类型", "测量量程", "测量精度", "测量间隔", "消解温度", "消解时长", "空白校准时间", "曲线截距", "曲线斜率", "测量检出限", "测量信号值", "线性相关系数", "二次多项式系数", "标样校准时间"] ("columns输出")] -> w337
        tunnel: w335 -> [w365 _]
        frame "STD" {
          n130 = case shown="\"CODMn\"" w365 {
            tunnel: [string[] ["时间", "数据类型", "测量量程", "测量精度", "测量间隔", "消解温度", "消解时长", "空白校准时间", "曲线截距", "曲线斜率", "测量检出限", "测量信号值", "线性相关系数", "二次多项式系数", "标样校准时间", "量程"] ("columns输出") string[] ["时间", "数据类型", "测量量程", "测量精度", "测量间隔", "消解温度", "消解时长", "空白校准时间", "曲线截距", "曲线斜率", "测量检出限", "测量信号值", "线性相关系数", "二次多项式系数", "标样校准时间", "量程标识"] ("columns输出")] -> w366
            frame "CODMn" {
            }
            frame "", Default {
            }
          }
        }
        frame "GB212", Default {
        }
      }
      n131 = call "数据库加密匹配 (子VI).vi"("输入参数"="N") -> ("Encoded String"=w340:string)  [unwired: 10 in]
      n132 = global read "全局 时间2.vi" "时间2"() -> (w349:string)
      n133 = global read "全局 水样时间.vi" "时间"() -> (w347:string)
      n134 = Format Into String(format string="where 数据类型 = '%s' and 时间 between" ("condition"), w340) -> (resulting string=w341:string)  [unwired: 2 in, 1 out]
      n135 = Format Into String(format string="#%s#" ("初始字符串"), w347) -> (resulting string=w354:string)  [unwired: 2 in, 1 out]
      n136 = Format Into String(format string="#%s#" ("初始字符串"), w349) -> (resulting string=w350:string)  [unwired: 2 in, 1 out]
      n137 = Concatenate Strings(w341, w354, "and" ("字符串"), w350, " order by 时间 desc" ("字符串")) -> (w346:string)
      n138 = call "SQL查询.vi"("condition"=w346, "columns"=w337, "table输入"=w335, "database"="database1.mdb") -> ("error out"=w343:errorcluster, "data"=w344:string[][])  [unwired: 4 in, 2 out]
      n139 = Empty Array?(array=w344) -> (empty?=w345:bool)
      n140 = case shown="真" w345 {
        tunnel: [w370 w386] -> w364
        tunnel: w338 -> [_ w374]
        tunnel: [w371 w372] -> w363
        tunnel: w344 -> [w371 _]
        tunnel: w343 -> [w370 _]
        frame False {
        }
        frame True {
          n141 = global read "全局 时间2.vi" "时间2"() -> (w379:string)
          n142 = global read "全局 水样时间.vi" "时间"() -> (w373:string)
          n143 = Format Into String(format string="where 参数 = '%s' and 时间 between" ("condition"), w374) -> (resulting string=w378:string)  [unwired: 2 in, 1 out]
          n144 = Format Into String(format string="#%s#" ("初始字符串"), w373) -> (resulting string=w384:string)  [unwired: 2 in, 1 out]
          n145 = Format Into String(format string="#%s#" ("初始字符串"), w379) -> (resulting string=w380:string)  [unwired: 2 in, 1 out]
          n146 = Concatenate Strings(w378, w384, "and" ("字符串"), w380, " order by 时间 desc" ("字符串")) -> (w385:string)
          n147 = call "SQL查询.vi"("condition"=w385, "table输入"="仪器参数", "database"="database3.mdb") -> ("error out"=w386:errorcluster, "data"=w372:string[][])  [unwired: 5 in, 2 out]
        }
      }
      n148 = Get Date/Time In Seconds() -> (seconds since 1Jan1904=w360:timestamp)
      n149 = Format Date/Time String(time format string (%c)="%Y/%m/%d %H:%M:%S" ("时间格式字符串(%c)"), seconds (now)=w360) -> (date/time string=w361:string)  [unwired: 1 in]
      n150 = Search and Replace String(input string=w361, search string="." ("搜索字符串")) -> (result string=w357:string)  [unwired: 6 in, 3 out]
      n151 = Replace Array Subset(array=w363, new element=w357, index (row)=w358, index (col)=w358) -> (w356:string[][])
    }
    frame "报警信息", "报警信息存表" {
      # "时间"
      n152 = case shown="\"报警信息\", \"报警信息存表\", \"操作日志\", \"系统状态\"" w393 {
        tunnel: ["database1.mdb" ("database") "database3.mdb" ("database")] -> w404
        frame Default {
        }
        frame "报警信息", "报警信息存表", "操作日志", "系统状态" {
        }
      }
      n153 = case shown="\"环境参数\"" w393 {
        tunnel: [w454 "报警信息" ("table输入")] -> w394
        frame "环境参数" {
          n154 = local read "仪器日志参数"() -> (w454:string)
        }
        frame "报警信息", Default {
        }
      }
      n155 = case shown="\"环境参数\"" w389 {
        tunnel: [" order by 时间 desc" ("字符串") "" ("仪器日志参数")] -> w392
        frame "环境参数" {
        }
        frame "报警信息", Default {
        }
      }
      n156 = case shown="\"报警信息\"" w389 {
        tunnel: [w406 w409] -> w390
        tunnel: [w405 w408] -> w391
        tunnel: w388 -> [_ w410]
        frame "", Default {
          n157 = global read "全局 时间2.vi" "时间2"() -> (w405:string)
          n158 = global read "全局 水样时间.vi" "时间"() -> (w406:string)
        }
        frame "报警信息" {
          n159 = global read "全局 时间2.vi" "报警信息索引"() -> (w407:T3)
          n160 = case shown="\"氟化物\"" w410 {
            tunnel: [w411 w415 w418 w421 w424 w427 w430 w433 w436 w439 w442 w445 w448 w451] -> w408
            tunnel: [w412 w414 w416 w419 w422 w425 w428 w431 w434 w437 w440 w443 w446 w449] -> w409
            tunnel: w407 -> [_ w413 w417 w420 w423 w426 w429 w432 w435 w438 w441 w444 w447 w450]
            frame "假", Default {
              n161 = global read "全局 时间2.vi" "时间2"() -> (w411:string)
              n162 = global read "全局 水样时间.vi" "时间"() -> (w412:string)
            }
            frame "CODMn" {
              n163 = Unbundle By Name(w413) -> ("CODMn报警信息索引起始时间"=w414:string)
              n164 = global read "全局 时间2.vi" "时间2"() -> (w415:string)
            }
            frame "氨氮" {
              n165 = Unbundle By Name(w417) -> ("氨氮报警信息索引起始时间"=w416:string)
              n166 = global read "全局 时间2.vi" "时间2"() -> (w418:string)
            }
            frame "总磷" {
              n167 = Unbundle By Name(w420) -> ("总磷报警信息索引起始时间"=w419:string)
              n168 = global read "全局 时间2.vi" "时间2"() -> (w421:string)
            }
            frame "总氮" {
              n169 = Unbundle By Name(w423) -> ("总氮报警信息索引起始时间"=w422:string)
              n170 = global read "全局 时间2.vi" "时间2"() -> (w424:string)
            }
            frame "CODCr" {
              n171 = Unbundle By Name(w426) -> ("CODCr报警信息索引起始时间"=w425:string)
              n172 = global read "全局 时间2.vi" "时间2"() -> (w427:string)
            }
            frame "DO" {
              n173 = Unbundle By Name(w429) -> ("DO报警信息索引起始时间"=w428:string)
              n174 = global read "全局 时间2.vi" "时间2"() -> (w430:string)
            }
            frame "PH" {
              n175 = Unbundle By Name(w432) -> ("PH报警信息索引起始时间"=w431:string)
              n176 = global read "全局 时间2.vi" "时间2"() -> (w433:string)
            }
            frame "电导率" {
              n177 = Unbundle By Name(w435) -> ("比电导率报警信息索引起始时间"=w434:string)
              n178 = global read "全局 时间2.vi" "时间2"() -> (w436:string)
            }
            frame "水温" {
              n179 = Unbundle By Name(w438) -> ("水温报警信息索引起始时间"=w437:string)
              n180 = global read "全局 时间2.vi" "时间2"() -> (w439:string)
            }
            frame "浊度" {
              n181 = Unbundle By Name(w441) -> ("浊度报警信息索引起始时间"=w440:string)
              n182 = global read "全局 时间2.vi" "时间2"() -> (w442:string)
            }
            frame "叶绿素" {
              n183 = Unbundle By Name(w444) -> ("叶绿素报警信息索引起始时间"=w443:string)
              n184 = global read "全局 时间2.vi" "时间2"() -> (w445:string)
            }
            frame "系统" {
              n185 = Unbundle By Name(w447) -> ("系统报警信息索引起始时间"=w446:string)
              n186 = global read "全局 时间2.vi" "时间2"() -> (w448:string)
            }
            frame "氟化物" {
              n187 = Unbundle By Name(w450) -> ("氟化物报警信息索引起始时间"=w449:string)
              n188 = global read "全局 时间2.vi" "时间2"() -> (w451:string)
            }
          }
        }
      }
      n189 = case shown="\"报警信息\", 默认" w389 {
        tunnel: [w458 w462 "where 时间 between" ("condition")] -> w395
        tunnel: w388 -> [w457 w461 _]
        frame "报警信息", Default {
          n190 = call "数据库加密匹配 (子VI).vi"("输入参数"=w457) -> ("Encoded String"=w456:string)  [unwired: 10 in]
          n191 = Format Into String(format string="where 参数 = '%s' and 时间 between" ("condition"), w456) -> (resulting string=w458:string)  [unwired: 2 in, 1 out]
        }
        frame "环境参数" {
          n192 = call "数据库加密匹配 (子VI).vi"("输入参数"=w461) -> ("Encoded String"=w460:string)  [unwired: 10 in]
          n193 = Format Into String(format string="where 参数 = '%s' and 时间 between" ("condition"), w460) -> (resulting string=w462:string)  [unwired: 2 in, 1 out]
        }
        frame "报警信息存表" {
        }
      }
      n194 = Format Into String(format string="#%s#" ("初始字符串"), w391) -> (resulting string=w396:string)  [unwired: 2 in, 1 out]
      n195 = Format Into String(format string="#%s#" ("初始字符串"), w390) -> (resulting string=w400:string)  [unwired: 2 in, 1 out]
      n196 = Concatenate Strings(w395, w400, "and" ("字符串"), w396, w392) -> (w402:string)
      n197 = call "SQL查询.vi"("condition"=w402, "table输入"=w394, "database"=w404) -> ("error out"=w403:errorcluster, "data"=w401:string[][])  [unwired: 5 in, 2 out]
    }
    frame "提取报警信息" {
      w472 = 0 ("索引 (行)")
      # "时间"
      # "提取仪器状态"
      n198 = call "数据库加密匹配 (子VI).vi"("输入参数"=w468) -> ("Encoded String"=w467:string)  [unwired: 10 in]
      n199 = global read "全局 水样时间.vi" "时间"() -> (w478:string)
      n200 = global read "全局 时间2.vi" "时间2"() -> (w479:string)
      n201 = Format Into String(format string="where 参数 = '%s' and 时间 between" ("condition"), w467) -> (resulting string=w482:string)  [unwired: 2 in, 1 out]
      n202 = Format Into String(format string="#%s#" ("初始字符串"), w478) -> (resulting string=w487:string)  [unwired: 2 in, 1 out]
      n203 = Format Into String(format string="#%s#" ("初始字符串"), w479) -> (resulting string=w483:string)  [unwired: 2 in, 1 out]
      n204 = Concatenate Strings(w482, w487, "and" ("字符串"), w483, " order by 时间 desc" ("仪器日志参数")) -> (w488:string)
      n205 = Get Date/Time In Seconds() -> (seconds since 1Jan1904=w474:timestamp)
      n206 = Format Date/Time String(time format string (%c)="%Y/%m/%d %H:%M:%S" ("时间格式字符串(%c)"), seconds (now)=w474) -> (date/time string=w475:string)  [unwired: 1 in]
      n207 = call "SQL查询.vi"("condition"=w488, "table输入"="报警信息", "database"="database3.mdb") -> ("error out"=w489:errorcluster, "data"=w470:string[][])  [unwired: 5 in, 2 out]
      n208 = Search and Replace String(input string=w475, search string="." ("搜索字符串")) -> (result string=w471:string)  [unwired: 6 in, 3 out]
      n209 = Replace Array Subset(array=w470, new element=w471, index (row)=w472, index (col)=w472) -> (w469:string[][])
    }
    frame "环境参数" {
      n210 = call "SQL查询.vi"("condition"=" order by 时间 desc" ("字符串"), "columns"=string[] ["时间", "电压", "室温", "湿度", "GPS经度", "GPS纬度"] ("columns输出 2"), "table输入"=w493, "database"="database1.mdb") -> ("error out"=w497:errorcluster, "columns输出"=w492:string[], "data"=w496:string[][])  [unwired: 4 in, 1 out]
    }
    frame Default {
      # "时间格式转换"
      n211 = local read "待发送数据"() -> (w499:string[][])
      n212 = call "数组时间戳格式化(子VI).vi"("待发送数据输入"=w499) -> ("待发送数据输出"=w498:string[][])  [unwired: 10 in]
    }
    frame "实时数据" {
      (unwired) " order by 时间 desc" ("字符串")
      w506 = "database1.mdb" ("database")
      # "上传本地时间点的实时数据"
      # "上传质控数据（空白测试，跨度核查，核查数据，平行样数据）"
      n213 = global read "全局 实时数据参数.vi" "实时数据参数"() -> (w502:string)
      n214 = case shown="\"水样测试\"" w502 {
        tunnel: [w557 w583 w608 w647] -> w521
        tunnel: w502 -> [w554 w578 _ w644]
        tunnel: [w555 w579 w605 w645] -> w517
        tunnel: w507 -> [_ w582 _ _]
        frame "水样测试" {
          n215 = call "数据库加密匹配 (子VI).vi"("输入参数"=w554) -> ("Encoded String"=w553:string)  [unwired: 10 in]
          n216 = call "数据库加密匹配 (子VI).vi"("输入参数"="N") -> ("Encoded String"=w551:string)  [unwired: 10 in]
          n217 = Get Date/Time In Seconds() -> (seconds since 1Jan1904=w565:timestamp)
          n218 = Format Date/Time String(time format string (%c)="%Y%m%d%H%M%S%3u" ("时间格式字符串(%c)"), seconds (now)=w565) -> (date/time string=w563:string)  [unwired: 1 in]
          n219 = local read "查询元素输入"() -> (w558:string)
          n220 = Replace Substring(2:8 ("长度（子字符串长度）"), 3:10 ("偏移量(0)"), 4:"0000" ("子字符串(\"\")"), 5:w563) -> (1:w559:string)  [unwired: 1 out]
          n221 = case shown="\"CODCr加标回收率\", \"CODMn加标回收率\", \"氨氮加标回收率\", \"总氮加标回收率\", \"总磷加标回收率\"" w558 {
            tunnel: w559 -> [w567 w570 _]
            tunnel: [w566 w571 w572] -> w557
            frame Default {
              n222 = Search and Replace String(input string=w567, search string="." ("搜索字符串")) -> (result string=w568:string)  [unwired: 6 in, 3 out]
              n223 = call "格式时间字符串.vi"("字符串"=w568) -> ("连接的字符串"=w566:string)  [unwired: 10 in]
            }
            frame "CODCr", "CODMn", "累积流量", "总氮", "总磷" {
              n224 = call "实时数据查询用2小时间的数据.vi"("字符串"=w570) -> ("连接的字符串"=w571:string)  [unwired: 10 in]
            }
            frame "CODCr加标回收率", "CODMn加标回收率", "氨氮加标回收率", "总氮加标回收率", "总磷加标回收率" {
              n225 = global read "全局 时间2.vi" "加标回收索引起始时间"() -> (w572:string)
            }
          }
          n226 = Format Into String(format string="where 测量模式 ='%s' and 数据类型 ='%s' and 时间 > " ("格式字符串"), w553, w551) -> (resulting string=w555:string)  [unwired: 2 in, 1 out]
        }
        frame "空白测试" {
          n227 = call "数据库加密匹配 (子VI).vi"("输入参数"=w578) -> ("Encoded String"=w577:string)  [unwired: 10 in]
          n228 = global read "全局 时间2.vi" "零点核查索引"() -> (w581:T4)
          n229 = case shown="\"硫化物\"" w582 {
            tunnel: [w584 w586 w588 w590 w592 w595 w596 w598 w600] -> w583
            tunnel: w581 -> [w585 w587 w589 w591 w593 w594 w597 w599 _]
            frame "CODMn" {
              n230 = Unbundle By Name(w585) -> ("CODMn零点核查索引起始时间"=w584:string)
            }
            frame "CODCr" {
              n231 = Unbundle By Name(w587) -> ("CODCr零点核查索引起始时间"=w586:string)
            }
            frame "氨氮" {
              n232 = Unbundle By Name(w589) -> ("氨氮零点核查索引起始时间"=w588:string)
            }
            frame "总磷" {
              n233 = Unbundle By Name(w591) -> ("总磷零点核查索引起始时间"=w590:string)
            }
            frame "总氮" {
              n234 = Unbundle By Name(w593) -> ("总氮零点核查索引起始时间"=w592:string)
            }
            frame "亚硝酸盐" {
              n235 = Unbundle By Name(w594) -> ("亚硝酸盐零点核查索引起始时间"=w595:string)
            }
            frame "硫化物" {
              n236 = Unbundle By Name(w597) -> ("硫化物零点核查索引起始时间"=w596:string)
            }
            frame "ORP" {
              n237 = Unbundle By Name(w599) -> ("ORP零点核查索引起始时间"=w598:string)
            }
            frame "", Default {
              n238 = global read "全局 时间2.vi" "零点核查索引起始时间"() -> (w600:string)
            }
          }
          n239 = call "数据库加密匹配 (子VI).vi"("输入参数"="零点核查") -> ("Encoded String"=w575:string)  [unwired: 10 in]
          n240 = call "数据库加密匹配 (子VI).vi"("输入参数"="M") -> ("Encoded String"=w573:string)  [unwired: 10 in]
          n241 = Format Into String(format string="where (测量模式 ='%s'' or 测量模式 = '%s') and 数据类型 <>'%s' and 时间 > " ("格式字符串"), w577, w575, w573) -> (resulting string=w579:string)  [unwired: 2 in, 1 out]
        }
        frame "核查数据" {
          n242 = global read "全局 时间2.vi" "标样核查索引"() -> (w607:T5)
          n243 = local read "查询元素输入"() -> (w609:string)
          n244 = case shown="\"ORP\"" w609 {
            tunnel: [w610 w612 w614 w616 w618 w620 w622 w624 w626 w628 w630 w632 w634 w636 w638 w640] -> w608
            tunnel: w607 -> [w611 w613 w615 w617 w619 w621 w623 w625 w627 w629 w631 w633 w635 w637 w639 _]
            frame "CODMn" {
              n245 = Unbundle By Name(w611) -> ("CODMn标样核查索引起始时间"=w610:string)
            }
            frame "CODCr" {
              n246 = Unbundle By Name(w613) -> ("CODCr标样核查索引起始时间"=w612:string)
            }
            frame "氨氮" {
              n247 = Unbundle By Name(w615) -> ("氨氮标样核查索引起始时间"=w614:string)
            }
            frame "总磷" {
              n248 = Unbundle By Name(w617) -> ("总磷标样核查索引起始时间"=w616:string)
            }
            frame "总氮" {
              n249 = Unbundle By Name(w619) -> ("总氮标样核查索引起始时间"=w618:string)
            }
            frame "DO" {
              n250 = Unbundle By Name(w621) -> ("DO标样核查索引起始时间"=w620:string)
            }
            frame "PH" {
              n251 = Unbundle By Name(w623) -> ("PH标样核查索引起始时间"=w622:string)
            }
            frame "比电导率" {
              n252 = Unbundle By Name(w625) -> ("比电导率标样核查索引起始时间"=w624:string)
            }
            frame "水温" {
              n253 = Unbundle By Name(w627) -> ("水温标样核查索引起始时间"=w626:string)
            }
            frame "浊度" {
              n254 = Unbundle By Name(w629) -> ("浊度标样核查索引起始时间"=w628:string)
            }
            frame "叶绿素a" {
              n255 = Unbundle By Name(w631) -> ("叶绿素a标样核查索引起始时间"=w630:string)
            }
            frame "藻密度" {
              n256 = Unbundle By Name(w633) -> ("藻密度标样核查索引起始时间"=w632:string)
            }
            frame "亚硝酸盐" {
              n257 = Unbundle By Name(w635) -> ("亚硝酸盐标样核查索引起始时间"=w634:string)
            }
            frame "硫化物" {
              n258 = Unbundle By Name(w637) -> ("硫化物标样核查索引起始时间"=w636:string)
            }
            frame "ORP" {
              n259 = Unbundle By Name(w639) -> ("ORP标样核查索引起始时间"=w638:string)
            }
            frame "", Default {
              n260 = global read "全局 时间2.vi" "标样核查索引起始时间"() -> (w640:string)
            }
          }
          n261 = call "数据库加密匹配 (子VI).vi"("输入参数"="标样核查" ("实时数据参数")) -> ("Encoded String"=w601:string)  [unwired: 10 in]
          n262 = call "数据库加密匹配 (子VI).vi"("输入参数"="M") -> ("Encoded String"=w603:string)  [unwired: 10 in]
          n263 = Format Into String(format string="where 测量模式 ='%s' and 数据类型 <> '%s' and 时间 > " ("格式字符串"), w601, w603) -> (resulting string=w605:string)  [unwired: 2 in, 1 out]
        }
        frame "跨度核查", Default {
          n264 = call "数据库加密匹配 (子VI).vi"("输入参数"=w644) -> ("Encoded String"=w643:string)  [unwired: 10 in]
          n265 = call "数据库加密匹配 (子VI).vi"("输入参数"="M") -> ("Encoded String"=w641:string)  [unwired: 10 in]
          n266 = global read "全局 时间2.vi" "跨度核查索引"() -> (w649:T6)
          n267 = local read "查询元素输入"() -> (w648:string)
          n268 = case shown="\"氨氮\"" w648 {
            tunnel: [w650 w652 w654 w656 w658 w661 w662 w664 w666] -> w647
            tunnel: w649 -> [w651 w653 w655 w657 w659 w660 w663 w665 _]
            frame "CODMn" {
              n269 = Unbundle By Name(w651) -> ("CODMn跨度核查索引起始时间"=w650:string)
            }
            frame "CODCr" {
              n270 = Unbundle By Name(w653) -> ("CODCr跨度核查索引起始时间"=w652:string)
            }
            frame "氨氮" {
              n271 = Unbundle By Name(w655) -> ("氨氮跨度核查索引起始时间"=w654:string)
            }
            frame "总磷" {
              n272 = Unbundle By Name(w657) -> ("总磷跨度核查索引起始时间"=w656:string)
            }
            frame "总氮" {
              n273 = Unbundle By Name(w659) -> ("总氮跨度核查索引起始时间"=w658:string)
            }
            frame "亚硝酸盐" {
              n274 = Unbundle By Name(w660) -> ("亚硝酸盐跨度核查索引起始时间"=w661:string)
            }
            frame "硫化物" {
              n275 = Unbundle By Name(w663) -> ("硫化物跨度核查索引起始时间"=w662:string)
            }
            frame "ORP" {
              n276 = Unbundle By Name(w665) -> ("ORP跨度核查索引起始时间"=w664:string)
            }
            frame "", Default {
              n277 = global read "全局 时间2.vi" "跨度核查索引起始时间"() -> (w666:string)
            }
          }
          n278 = Format Into String(format string="where 测量模式 ='%s' and 数据类型 <> '%s' and 时间 > " ("格式字符串"), w643, w641) -> (resulting string=w645:string)  [unwired: 2 in, 1 out]
        }
      }
      n279 = case shown="\"假\", 默认" w502 {
        tunnel: [string[] ["时间", "测量模式", "数据类型", "检测值", "单位", "数据标识", "标样参考值"] ("columns") string[] ["时间", "测量模式", "数据类型", "检测值", "单位", "数据标识", "标样参考值", "跨度值"] ("columns")] -> w512
        frame "假", Default {
        }
        frame "空白测试", "跨度核查" {
        }
      }
      n280 = global read "断电保存全局.vi" "数据发送延时时间/s"() -> (w511:i32)
      n281 = Get Date/Time In Seconds() -> (seconds since 1Jan1904=w510:timestamp)
      n282 = Subtract(x=w510, y=w511) -> (x-y=w509:timestamp)
      n283 = global read "断电保存全局.vi" "数据组合发送"() -> (w514:bool)
      n284 = Seconds To Date/Time(time stamp (now)=w509) -> (date time rec=w516:T7)  [unwired: 1 in]
      n285 = case shown="真" w514 {
        tunnel: w516 -> [w545 w550]
        tunnel: [w545 w549] -> w515
        frame False {
        }
        frame True {
          n286 = Unbundle By Name(w550) -> ("时"=w548:i32)
          n287 = Subtract(x=w548, y=2) -> (x-y=w546:i32)
          n288 = Bundle By Name(cluster=w550, "时"=w546) -> (w549:T7)
        }
      }
      n289 = Date/Time To Seconds(2:w515) -> (0:w520:timestamp)  [unwired: 1 in]
      n290 = Format Date/Time String(time format string (%c)="%Y/%m/%d %H:%M:%S" ("时间格式字符串(%c)"), seconds (now)=w520) -> (date/time string=w518:string)  [unwired: 1 in]
      n291 = Format Into String(format string="#%s#" ("初始字符串"), w521) -> (resulting string=w526:string)  [unwired: 2 in, 1 out]
      n292 = Format Into String(format string="#%s#" ("初始字符串"), w518) -> (resulting string=w523:string)  [unwired: 2 in, 1 out]
      n293 = Concatenate Strings(w517, w526, "and 时间 < " ("字符串"), w523, " order by 时间 asc" ("字符串")) -> (w505:string)
      n294 = call "SQL查询.vi"("condition"=w505, "columns"=w512, "table输入"=w507, "database"=w506) -> ("error out"=w508:errorcluster, "data"=w504:string[][])  [unwired: 4 in, 2 out]
      n295 = case shown="错误" w508 {
        selector: w508 -> [w527 _]
        tunnel: w502 -> [_ w535]
        tunnel: w507 -> [_ w534]
        tunnel: w506 -> [_ w533]
        tunnel: w505 -> [_ w532]
        tunnel: w504 -> [w528 w530]
        tunnel: [w528 w531] -> w503
        tunnel: [w527 w529] -> w501
        frame No Error {
        }
        frame Error {
          # "兼容旧数据库没有跨度值版本"
          n296 = case shown="\"空白测试\", \"跨度核查\"" w535 {
            tunnel: w534 -> [_ w541]
            tunnel: w533 -> [_ w540]
            tunnel: w532 -> [_ w539]
            tunnel: [w536 w538] -> w531
            tunnel: w530 -> [w536 _]
            tunnel: [_ w537] -> w529
            frame "假", Default {
            }
            frame "空白测试", "跨度核查" {
              n297 = call "SQL查询.vi"("condition"=w539, "columns"=string[] ["时间", "测量模式", "数据类型", "检测值", "单位", "数据标识", "标样参考值"], "table输入"=w541, "database"=w540) -> ("error out"=w537:errorcluster, "data"=w538:string[][])  [unwired: 4 in, 2 out]
            }
          }
        }
      }
      n298 = case shown="默认" w507 {
        tunnel: w507 -> [_ w669]
        tunnel: w505 -> [_ w668]
        tunnel: w503 -> [_ w667]
        frame Default {
        }
        frame "CODCr", "总氮", "总磷" {
          n299 = global write "全局 实时数据参数.vi" "data"(w667) -> ()
          n300 = global write "全局 实时数据参数.vi" "参数"(w669) -> ()
          n301 = global write "全局 实时数据参数.vi" "连接的字符串"(w668) -> ()
        }
      }
    }
    frame "加标回收" {
      w681 = "加标回收率" ("字符串")
      # "上传加标回收数据"
      n302 = call "数据库加密匹配 (子VI).vi"("输入参数"=w671) -> ("Encoded String"=w670:string)  [unwired: 10 in]
      n303 = global read "全局 数据发送重叠.vi" "掉线指示灯"() -> (w682:bool)
      n304 = case shown="假" w682 {
        tunnel: [w696 w711] -> w683
        frame False {
          n305 = global read "全局 时间2.vi" "加标回收索引"() -> (w702:T8)
          n306 = Unbundle By Name(w702) -> ("氨氮加标回收索引起始时间"=w701:string, "总磷加标回收索引起始时间"=w700:string, "总氮加标回收索引起始时间"=w699:string, "CODMn加标回收索引起始时间"=w698:string, "CODCr加标回收索引起始时间"=w697:string, "氟化物加标回收索引起始时间"=w695:string)
          n307 = local read "查询元素输入"() -> (w703:string)
          n308 = case shown="\"氟化物加标回收率\"" w703 {
            tunnel: [w704 w705 w706 w707 w708 w709 w710] -> w696
            tunnel: w701 -> [_ _ w706 _ _ _ _]
            tunnel: w700 -> [_ _ _ w707 _ _ _]
            tunnel: w699 -> [_ _ _ _ w708 _ _]
            tunnel: w698 -> [w704 _ _ _ _ _ _]
            tunnel: w697 -> [_ w705 _ _ _ _ _]
            tunnel: w695 -> [_ _ _ _ _ w709 _]
            frame "CODMn加标回收率" {
            }
            frame "CODCr加标回收率" {
            }
            frame "氨氮加标回收率" {
            }
            frame "总磷加标回收率" {
            }
            frame "总氮加标回收率" {
            }
            frame "氟化物加标回收率" {
            }
            frame "", Default {
              n309 = global read "全局 时间2.vi" "加标回收索引起始时间"() -> (w710:string)
            }
          }
        }
        frame True {
          n310 = global read "全局 数据发送重叠.vi" "TCP掉线时间节点"() -> (w711:string)
        }
      }
      n311 = global read "断电保存全局.vi" "数据发送延时时间/s"() -> (w674:i32)
      n312 = Get Date/Time In Seconds() -> (seconds since 1Jan1904=w673:timestamp)
      n313 = Subtract(x=w673, y=w674) -> (x-y=w672:timestamp)
      n314 = Seconds To Date/Time(time stamp (now)=w672) -> (date time rec=w678:T7)  [unwired: 1 in]
      n315 = Date/Time To Seconds(2:w678) -> (0:w680:timestamp)  [unwired: 1 in]
      n316 = Format Date/Time String(time format string (%c)="%Y/%m/%d %H:%M:%S" ("时间格式字符串(%c)"), seconds (now)=w680) -> (date/time string=w677:string)  [unwired: 1 in]
      n317 = Format Into String(format string="#%s#" ("初始字符串"), w683) -> (resulting string=w694:string)  [unwired: 2 in, 1 out]
      n318 = Format Into String(format string="#%s#" ("初始字符串"), w677) -> (resulting string=w690:string)  [unwired: 2 in, 1 out]
      n319 = Concatenate Strings("where 参数 ='" ("condition"), w670, "' and 时间 > ", w694, "and 时间 < " ("字符串"), w690, " order by 时间 asc" ("字符串")) -> (w685:string)
      n320 = call "SQL查询.vi"("condition"=w685, "columns"=string[] ["时间", "参数", "加标前水样测试时间", "加标前水样浓度值", "加标后水样浓度值", "加标母液浓度值", "加标体积", "加标水杯定容体积", "加标回收率"], "table输入"=w681, "database"="database1.mdb") -> ("error out"=w686:errorcluster, "data"=w684:string[][])  [unwired: 4 in, 2 out]
      n321 = case shown="默认" w681 {
        tunnel: w681 -> [_ w714]
        tunnel: w685 -> [_ w713]
        tunnel: w684 -> [_ w712]
        frame Default {
        }
        frame "CODCr", "总氮", "总磷" {
          n322 = global write "全局 实时数据参数.vi" "data"(w712) -> ()
          n323 = global write "全局 实时数据参数.vi" "参数"(w714) -> ()
          n324 = global write "全局 实时数据参数.vi" "连接的字符串"(w713) -> ()
        }
      }
    }
    frame "平行样测试" {
      w726 = "平行样测试" ("字符串")
      # "上传本地时间点的实时数据"
      # "上传平行样数据"
      n325 = call "数据库加密匹配 (子VI).vi"("输入参数"=w716) -> ("Encoded String"=w715:string)  [unwired: 10 in]
      n326 = global read "全局 数据发送重叠.vi" "掉线指示灯"() -> (w727:bool)
      n327 = case shown="假" w727 {
        tunnel: [w751 w759] -> w728
        frame False {
          n328 = global read "全局 时间2.vi" "平行样索引"() -> (w749:T9)
          n329 = Unbundle By Name(w749) -> ("氨氮平行样索引起始时间"=w748:string, "总磷平行样索引起始时间"=w747:string, "总氮平行样索引起始时间"=w746:string, "CODMn平行样索引起始时间"=w745:string, "CODCr平行样索引起始时间"=w744:string, "氟化物平行样索引起始时间"=w743:string)
          n330 = local read "查询元素输入"() -> (w750:string)
          n331 = case shown="\"氟化物\"" w750 {
            tunnel: [w752 w753 w754 w755 w756 w757 w758] -> w751
            tunnel: w748 -> [_ _ w754 _ _ _ _]
            tunnel: w747 -> [_ _ _ w755 _ _ _]
            tunnel: w746 -> [_ _ _ _ w756 _ _]
            tunnel: w745 -> [w752 _ _ _ _ _ _]
            tunnel: w744 -> [_ w753 _ _ _ _ _]
            tunnel: w743 -> [_ _ _ _ _ w757 _]
            frame "CODMn" {
            }
            frame "CODCr" {
            }
            frame "氨氮" {
            }
            frame "总磷" {
            }
            frame "总氮" {
            }
            frame "氟化物" {
            }
            frame "", Default {
              n332 = global read "全局 时间2.vi" "平行样索引起始时间"() -> (w758:string)
            }
          }
        }
        frame True {
          n333 = global read "全局 数据发送重叠.vi" "TCP掉线时间节点"() -> (w759:string)
        }
      }
      n334 = global read "断电保存全局.vi" "数据发送延时时间/s"() -> (w719:i32)
      n335 = Get Date/Time In Seconds() -> (seconds since 1Jan1904=w718:timestamp)
      n336 = Subtract(x=w718, y=w719) -> (x-y=w717:timestamp)
      n337 = Seconds To Date/Time(time stamp (now)=w717) -> (date time rec=w723:T7)  [unwired: 1 in]
      n338 = Date/Time To Seconds(2:w723) -> (0:w725:timestamp)  [unwired: 1 in]
      n339 = Format Date/Time String(time format string (%c)="%Y/%m/%d %H:%M:%S" ("时间格式字符串(%c)"), seconds (now)=w725) -> (date/time string=w722:string)  [unwired: 1 in]
      n340 = Format Into String(format string="#%s#" ("初始字符串"), w728) -> (resulting string=w742:string)  [unwired: 2 in, 1 out]
      n341 = Format Into String(format string="#%s#" ("初始字符串"), w722) -> (resulting string=w738:string)  [unwired: 2 in, 1 out]
      n342 = Concatenate Strings("where 参数 ='" ("condition"), w715, "' and 时间 > ", w742, "and 时间 < " ("字符串"), w738, " order by 时间 asc" ("字符串")) -> (w730:string)
      n343 = call "SQL查询.vi"("condition"=w730, "columns"=string[] ["时间", "参数", "第一次水样浓度值", "第二次水样测试时间", "第二次水样浓度值"], "table输入"=w726, "database"="database1.mdb") -> ("error out"=w732:errorcluster, "data"=w729:string[][])  [unwired: 4 in, 2 out]
      n344 = case shown="默认" w726 {
        tunnel: w726 -> [_ w762]
        tunnel: w730 -> [_ w761]
        tunnel: w729 -> [_ w760]
        frame Default {
        }
        frame "CODCr", "总氮", "总磷" {
          n345 = global write "全局 实时数据参数.vi" "data"(w760) -> ()
          n346 = global write "全局 实时数据参数.vi" "参数"(w762) -> ()
          n347 = global write "全局 实时数据参数.vi" "连接的字符串"(w761) -> ()
        }
      }
      n348 = case shown="假" FALSE {
        tunnel: [w764 w767] -> w734
        tunnel: w729 -> [w764 w766]
        tunnel: w732 -> [w763 w765]
        tunnel: [w763 w765] -> w731
        frame False {
        }
        frame True {
          # "数字字符串精度转换保留"
          n349 = Index Array(array=w766, index (col)=3 ("禁用的索引 (列)")) -> (element=w773:string[])  [unwired: 1 in]
          n350 = for {
            tunnel: w773 -> [w776] mode=indexing
            tunnel: [w775] -> w769 mode=indexing
            n351 = Fract/Exp String To Number(string=w776) -> (number=w777:dbl)  [unwired: 3 in, 1 out]
            n352 = Number To Fractional String(number=w777, precision (6)=i16 2 ("精度(6)")) -> (F-format string=w775:string)  [unwired: 2 in]
          }
          n353 = Delete From Array(array=w766, length=1 ("长度"), index (col)=3 ("禁用的索引 (列)")) -> (array with subset deleted=w770:string[][])  [unwired: 1 in, 1 out]
          n354 = Insert Into Array(array=w770, index (col)=3 ("禁用的索引 (列)"), new element=w769) -> (w767:string[][])  [unwired: 1 in]
        }
      }
    }
    frame "集成干预测试" {
      # "上传本地时间点的实时数据"
      # "上传集成干预数据"
      n355 = global read "全局 数据发送重叠.vi" "掉线指示灯"() -> (w792:bool)
      n356 = case shown="假" w792 {
        tunnel: [w816 w852] -> w793
        frame False {
          n357 = global read "全局 时间2.vi" "集成干预索引"() -> (w818:T10)
          n358 = local read "查询元素输入"() -> (w817:string)
          n359 = case shown="\"氟化物\"" w817 {
            tunnel: [w819 w821 w823 w825 w827 w829 w831 w833 w835 w837 w839 w841 w843 w845 w847 w849 w851] -> w816
            tunnel: w818 -> [w820 w822 w824 w826 w828 w830 w832 w834 w836 w838 w840 w842 w844 w846 w848 w850 _]
            frame "CODMn" {
              n360 = Unbundle By Name(w820) -> ("CODMn集成干预索引起始时间"=w819:string)
            }
            frame "CODCr" {
              n361 = Unbundle By Name(w822) -> ("CODCr集成干预索引起始时间"=w821:string)
            }
            frame "氨氮" {
              n362 = Unbundle By Name(w824) -> ("氨氮集成干预索引起始时间"=w823:string)
            }
            frame "总磷" {
              n363 = Unbundle By Name(w826) -> ("总磷集成干预索引起始时间"=w825:string)
            }
            frame "总氮" {
              n364 = Unbundle By Name(w828) -> ("总氮集成干预索引起始时间"=w827:string)
            }
            frame "DO" {
              n365 = Unbundle By Name(w830) -> ("DO集成干预索引起始时间"=w829:string)
            }
            frame "PH" {
              n366 = Unbundle By Name(w832) -> ("PH集成干预索引起始时间"=w831:string)
            }
            frame "比电导率" {
              n367 = Unbundle By Name(w834) -> ("比电导率集成干预索引起始时间"=w833:string)
            }
            frame "水温" {
              n368 = Unbundle By Name(w836) -> ("水温集成干预索引起始时间"=w835:string)
            }
            frame "浊度" {
              n369 = Unbundle By Name(w838) -> ("浊度集成干预索引起始时间"=w837:string)
            }
            frame "叶绿素a" {
              n370 = Unbundle By Name(w840) -> ("叶绿素a集成干预索引起始时间"=w839:string)
            }
            frame "藻密度" {
              n371 = Unbundle By Name(w842) -> ("藻密度集成干预索引起始时间"=w841:string)
            }
            frame "亚硝酸盐" {
              n372 = Unbundle By Name(w844) -> ("亚硝酸盐集成干预索引起始时间"=w843:string)
            }
            frame "硫化物" {
              n373 = Unbundle By Name(w846) -> ("硫化物集成干预索引起始时间"=w845:string)
            }
            frame "ORP" {
              n374 = Unbundle By Name(w848) -> ("ORP集成干预索引起始时间"=w847:string)
            }
            frame "氟化物" {
              n375 = Unbundle By Name(w850) -> ("氟化物集成干预索引起始时间"=w849:string)
            }
            frame "", Default {
              n376 = global read "全局 时间2.vi" "平行样索引起始时间"() -> (w851:string)
            }
          }
        }
        frame True {
          n377 = global read "全局 数据发送重叠.vi" "TCP掉线时间节点"() -> (w852:string)
        }
      }
      n378 = global read "断电保存全局.vi" "应用环境"() -> (w783:enum16{"STD", "GB212"})
      n379 = case shown="\"STD\", 默认" w783 {
        tunnel: w782 -> [w805 w815]
        tunnel: ["集成干预测试" ("字符串") w815] -> w781
        tunnel: [string[] ["时间", "参数", "集成干预测试浓度值", "集成干预前测试时间", "集成干预前测试浓度值"] ("columns") string[] ["时间", "测量模式", "数据类型", "检测值", "单位", "数据标识", "因子编码", "标样参考值"] ("columns")] -> w780
        tunnel: [w807 w814] -> w779
        frame "STD", Default {
          n380 = call "数据库加密匹配 (子VI).vi"("输入参数"=w805) -> ("Encoded String"=w804:string)  [unwired: 10 in]
          n381 = Concatenate Strings("where 参数 ='" ("condition"), w804) -> (w807:string)
        }
        frame "GB212" {
          n382 = call "数据库加密匹配 (子VI).vi"("输入参数"="集成干预测试" ("字符串")) -> ("Encoded String"=w810:string)  [unwired: 10 in]
          n383 = Concatenate Strings("where 测量模式 ='" ("condition"), w810) -> (w814:string)
        }
      }
      n384 = global read "断电保存全局.vi" "数据发送延时时间/s"() -> (w786:i32)
      n385 = Get Date/Time In Seconds() -> (seconds since 1Jan1904=w785:timestamp)
      n386 = Subtract(x=w785, y=w786) -> (x-y=w784:timestamp)
      n387 = Seconds To Date/Time(time stamp (now)=w784) -> (date time rec=w789:T7)  [unwired: 1 in]
      n388 = Date/Time To Seconds(2:w789) -> (0:w791:timestamp)  [unwired: 1 in]
      n389 = Format Date/Time String(time format string (%c)="%Y/%m/%d %H:%M:%S" ("时间格式字符串(%c)"), seconds (now)=w791) -> (date/time string=w788:string)  [unwired: 1 in]
      n390 = Format Into String(format string="#%s#" ("初始字符串"), w793) -> (resulting string=w803:string)  [unwired: 2 in, 1 out]
      n391 = Format Into String(format string="#%s#" ("初始字符串"), w788) -> (resulting string=w799:string)  [unwired: 2 in, 1 out]
      n392 = Concatenate Strings(w779, "' and 时间 > ", w803, "and 时间 < " ("字符串"), w799, " order by 时间 asc" ("字符串")) -> (w795:string)
      n393 = call "SQL查询.vi"("condition"=w795, "columns"=w780, "table输入"=w781, "database"="database1.mdb") -> ("error out"=w796:errorcluster, "data"=w794:string[][])  [unwired: 4 in, 2 out]
      n394 = case shown="\"CODCr\", \"总氮\", \"总磷\"" w781 {
        tunnel: w781 -> [_ w855]
        tunnel: w795 -> [_ w854]
        tunnel: w794 -> [_ w853]
        frame Default {
        }
        frame "CODCr", "总氮", "总磷" {
          n395 = global write "全局 实时数据参数.vi" "data"(w853) -> ()
          n396 = global write "全局 实时数据参数.vi" "参数"(w855) -> ()
          n397 = global write "全局 实时数据参数.vi" "连接的字符串"(w854) -> ()
        }
      }
    }
    frame "提取加标回收" {
      w860 = "加标回收率" ("字符串")
      # "上传本地时间点的实时数据"
      n398 = call "数据库加密匹配 (子VI).vi"("输入参数"=w857) -> ("Encoded String"=w856:string)  [unwired: 10 in]
      n399 = global read "全局 数据发送重叠.vi" "掉线指示灯"() -> (w861:bool)
      n400 = case shown="假" w861 {
        tunnel: [w877 w878] -> w862
        frame False {
          n401 = global read "起始时间.vi" "起始时间"() -> (w877:string)
        }
        frame True {
          n402 = global read "全局 数据发送重叠.vi" "TCP掉线时间节点"() -> (w878:string)
        }
      }
      n403 = global read "起始时间.vi" "结束时间"() -> (w859:string)
      n404 = Format Into String(format string="#%s#" ("初始字符串"), w862) -> (resulting string=w876:string)  [unwired: 2 in, 1 out]
      n405 = Format Into String(format string="#%s#" ("初始字符串"), w859) -> (resulting string=w872:string)  [unwired: 2 in, 1 out]
      n406 = Concatenate Strings("where 参数 ='" ("condition"), w856, "' and 时间 between ", w876, "and" ("字符串"), w872) -> (w864:string)
      n407 = call "SQL查询.vi"("condition"=w864, "columns"=string[] ["时间", "参数", "加标前水样测试时间", "加标前水样浓度值", "加标后水样浓度值", "加标母液浓度值", "加标体积", "加标水杯定容体积", "加标回收率"], "table输入"=w860, "database"="database1.mdb") -> ("error out"=w866:errorcluster, "data"=w863:string[][])  [unwired: 4 in, 2 out]
      n408 = case shown="\"CODCr\", \"总氮\", \"总磷\"" w860 {
        tunnel: w860 -> [_ w881]
        tunnel: w864 -> [_ w880]
        tunnel: w863 -> [_ w879]
        frame Default {
        }
        frame "CODCr", "总氮", "总磷" {
          n409 = global write "全局 实时数据参数.vi" "data"(w879) -> ()
          n410 = global write "全局 实时数据参数.vi" "参数"(w881) -> ()
          n411 = global write "全局 实时数据参数.vi" "连接的字符串"(w880) -> ()
        }
      }
      n412 = case shown="假" FALSE {
        tunnel: [w883 w886] -> w868
        tunnel: w863 -> [w883 w885]
        tunnel: w866 -> [w882 w884]
        tunnel: [w882 w884] -> w865
        frame False {
        }
        frame True {
          # "数字字符串精度转换保留"
          n413 = Index Array(array=w885, index (col)=3 ("禁用的索引 (列)")) -> (element=w892:string[])  [unwired: 1 in]
          n414 = for {
            tunnel: w892 -> [w895] mode=indexing
            tunnel: [w894] -> w888 mode=indexing
            n415 = Fract/Exp String To Number(string=w895) -> (number=w896:dbl)  [unwired: 3 in, 1 out]
            n416 = Number To Fractional String(number=w896, precision (6)=i16 2 ("精度(6)")) -> (F-format string=w894:string)  [unwired: 2 in]
          }
          n417 = Delete From Array(array=w885, length=1 ("长度"), index (col)=3 ("禁用的索引 (列)")) -> (array with subset deleted=w889:string[][])  [unwired: 1 in, 1 out]
          n418 = Insert Into Array(array=w889, index (col)=3 ("禁用的索引 (列)"), new element=w888) -> (w886:string[][])  [unwired: 1 in]
        }
      }
    }
    frame "提取平行样" {
      w902 = "平行样测试" ("字符串")
      # "上传本地时间点的实时数据"
      n419 = call "数据库加密匹配 (子VI).vi"("输入参数"=w899) -> ("Encoded String"=w898:string)  [unwired: 10 in]
      n420 = global read "全局 数据发送重叠.vi" "掉线指示灯"() -> (w903:bool)
      n421 = case shown="假" w903 {
        tunnel: [w919 w920] -> w904
        frame False {
          n422 = global read "起始时间.vi" "起始时间"() -> (w919:string)
        }
        frame True {
          n423 = global read "全局 数据发送重叠.vi" "TCP掉线时间节点"() -> (w920:string)
        }
      }
      n424 = global read "起始时间.vi" "结束时间"() -> (w901:string)
      n425 = Format Into String(format string="#%s#" ("初始字符串"), w904) -> (resulting string=w918:string)  [unwired: 2 in, 1 out]
      n426 = Format Into String(format string="#%s#" ("初始字符串"), w901) -> (resulting string=w914:string)  [unwired: 2 in, 1 out]
      n427 = Concatenate Strings("where 参数 ='" ("condition"), w898, "' and 时间 between ", w918, "and" ("字符串"), w914) -> (w906:string)
      n428 = call "SQL查询.vi"("condition"=w906, "columns"=string[] ["时间", "参数", "第一次水样浓度值", "第二次水样测试时间", "第二次水样浓度值"], "table输入"=w902, "database"="database1.mdb") -> ("error out"=w908:errorcluster, "data"=w905:string[][])  [unwired: 4 in, 2 out]
      n429 = case shown="\"CODCr\", \"总氮\", \"总磷\"" w902 {
        tunnel: w902 -> [_ w923]
        tunnel: w906 -> [_ w922]
        tunnel: w905 -> [_ w921]
        frame Default {
        }
        frame "CODCr", "总氮", "总磷" {
          n430 = global write "全局 实时数据参数.vi" "data"(w921) -> ()
          n431 = global write "全局 实时数据参数.vi" "参数"(w923) -> ()
          n432 = global write "全局 实时数据参数.vi" "连接的字符串"(w922) -> ()
        }
      }
      n433 = case shown="假" FALSE {
        tunnel: [w925 w928] -> w910
        tunnel: w905 -> [w925 w927]
        tunnel: w908 -> [w924 w926]
        tunnel: [w924 w926] -> w907
        frame False {
        }
        frame True {
          # "数字字符串精度转换保留"
          n434 = Index Array(array=w927, index (col)=3 ("禁用的索引 (列)")) -> (element=w934:string[])  [unwired: 1 in]
          n435 = for {
            tunnel: w934 -> [w937] mode=indexing
            tunnel: [w936] -> w930 mode=indexing
            n436 = Fract/Exp String To Number(string=w937) -> (number=w938:dbl)  [unwired: 3 in, 1 out]
            n437 = Number To Fractional String(number=w938, precision (6)=i16 2 ("精度(6)")) -> (F-format string=w936:string)  [unwired: 2 in]
          }
          n438 = Delete From Array(array=w927, length=1 ("长度"), index (col)=3 ("禁用的索引 (列)")) -> (array with subset deleted=w931:string[][])  [unwired: 1 in, 1 out]
          n439 = Insert Into Array(array=w931, index (col)=3 ("禁用的索引 (列)"), new element=w930) -> (w928:string[][])  [unwired: 1 in]
        }
      }
    }
    frame "提取集成干预" {
      # "上传本地时间点的实时数据"
      n440 = global read "断电保存全局.vi" "应用环境"() -> (w944:enum16{"STD", "GB212"})
      n441 = case shown="\"GB212\"" w944 {
        tunnel: w940 -> [w962 w972]
        tunnel: ["集成干预测试" ("字符串") w972] -> w942
        tunnel: [string[] ["时间", "参数", "集成干预测试浓度值", "集成干预前测试时间", "集成干预前测试浓度值"] ("columns") string[] ["时间", "测量模式", "数据类型", "检测值", "单位", "数据标识", "因子编码", "标样参考值"] ("columns")] -> w943
        tunnel: [w964 w971] -> w941
        frame "STD", Default {
          n442 = call "数据库加密匹配 (子VI).vi"("输入参数"=w962) -> ("Encoded String"=w961:string)  [unwired: 10 in]
          n443 = Concatenate Strings("where 参数 ='" ("condition"), w961) -> (w964:string)
        }
        frame "GB212" {
          n444 = call "数据库加密匹配 (子VI).vi"("输入参数"="集成干预测试" ("字符串")) -> ("Encoded String"=w967:string)  [unwired: 10 in]
          n445 = Concatenate Strings("where 测量模式 ='" ("condition"), w967) -> (w971:string)
        }
      }
      n446 = global read "全局 数据发送重叠.vi" "掉线指示灯"() -> (w946:bool)
      n447 = case shown="假" w946 {
        tunnel: [w973 w974] -> w947
        frame False {
          n448 = global read "起始时间.vi" "起始时间"() -> (w973:string)
        }
        frame True {
          n449 = global read "全局 数据发送重叠.vi" "TCP掉线时间节点"() -> (w974:string)
        }
      }
      n450 = global read "起始时间.vi" "结束时间"() -> (w945:string)
      n451 = Format Into String(format string="#%s#" ("初始字符串"), w947) -> (resulting string=w960:string)  [unwired: 2 in, 1 out]
      n452 = Format Into String(format string="#%s#" ("初始字符串"), w945) -> (resulting string=w956:string)  [unwired: 2 in, 1 out]
      n453 = Concatenate Strings(w941, "' and 时间 between ", w960, "and" ("字符串"), w956) -> (w949:string)
      n454 = call "SQL查询.vi"("condition"=w949, "columns"=w943, "table输入"=w942, "database"="database1.mdb") -> ("error out"=w951:errorcluster, "data"=w948:string[][])  [unwired: 4 in, 2 out]
      n455 = case shown="\"CODCr\", \"总氮\", \"总磷\"" w942 {
        tunnel: w942 -> [_ w977]
        tunnel: w949 -> [_ w976]
        tunnel: w948 -> [_ w975]
        frame Default {
        }
        frame "CODCr", "总氮", "总磷" {
          n456 = global write "全局 实时数据参数.vi" "data"(w975) -> ()
          n457 = global write "全局 实时数据参数.vi" "参数"(w977) -> ()
          n458 = global write "全局 实时数据参数.vi" "连接的字符串"(w976) -> ()
        }
      }
      n459 = case shown="假" FALSE {
        tunnel: [w979 w982] -> w953
        tunnel: w948 -> [w979 w981]
        tunnel: w951 -> [w978 w980]
        tunnel: [w978 w980] -> w950
        frame False {
        }
        frame True {
          # "数字字符串精度转换保留"
          n460 = Index Array(array=w981, index (col)=3 ("禁用的索引 (列)")) -> (element=w988:string[])  [unwired: 1 in]
          n461 = for {
            tunnel: w988 -> [w991] mode=indexing
            tunnel: [w990] -> w984 mode=indexing
            n462 = Fract/Exp String To Number(string=w991) -> (number=w992:dbl)  [unwired: 3 in, 1 out]
            n463 = Number To Fractional String(number=w992, precision (6)=i16 2 ("精度(6)")) -> (F-format string=w990:string)  [unwired: 2 in]
          }
          n464 = Delete From Array(array=w981, length=1 ("长度"), index (col)=3 ("禁用的索引 (列)")) -> (array with subset deleted=w985:string[][])  [unwired: 1 in, 1 out]
          n465 = Insert Into Array(array=w985, index (col)=3 ("禁用的索引 (列)"), new element=w984) -> (w982:string[][])  [unwired: 1 in]
        }
      }
    }
    frame "提取实时数据" {
      # "上传给定时间段之间的实时数据"
      n466 = global read "全局 实时数据参数.vi" "实时数据参数"() -> (w995:string)
      n467 = call "数据库加密匹配 (子VI).vi"("输入参数"=w995) -> ("Encoded String"=w994:string)  [unwired: 10 in]
      n468 = global read "起始时间.vi" "起始时间"() -> (w1006:string)
      n469 = global read "起始时间.vi" "结束时间"() -> (w1005:string)
      n470 = Format Into String(format string="#%s#" ("初始字符串"), w1006) -> (resulting string=w1013:string)  [unwired: 2 in, 1 out]
      n471 = Format Into String(format string="#%s#" ("初始字符串"), w1005) -> (resulting string=w1007:string)  [unwired: 2 in, 1 out]
      n472 = Concatenate Strings("where 测量模式 ='" ("condition"), w994, "' and 时间 between ", w1013, "and" ("字符串"), w1007) -> (w1011:string)
      n473 = call "SQL查询.vi"("condition"=w1011, "columns"=string[] ["时间", "测量模式", "数据类型", "检测值", "单位", "数据标识", "标样参考值"], "table输入"=w997, "database"="database1.mdb") -> ("error out"=w1002:errorcluster, "data"=w1004:string[][])  [unwired: 4 in, 2 out]
      n474 = case shown="假" FALSE {
        tunnel: w1004 -> [w1015 w1023]
        tunnel: [w1015 w1017] -> w1003
        tunnel: w1002 -> [w1014 w1016]
        tunnel: [w1014 w1016] -> w1001
        frame False {
        }
        frame True {
          # "数字字符串精度转换保留"
          n475 = Index Array(array=w1023, index (col)=3 ("禁用的索引 (列)")) -> (element=w1024:string[])  [unwired: 1 in]
          n476 = for {
            tunnel: w1024 -> [w1027] mode=indexing
            tunnel: [w1026] -> w1019 mode=indexing
            n477 = Fract/Exp String To Number(string=w1027) -> (number=w1028:dbl)  [unwired: 3 in, 1 out]
            n478 = Number To Fractional String(number=w1028, precision (6)=i16 2 ("精度(6)")) -> (F-format string=w1026:string)  [unwired: 2 in]
          }
          n479 = Delete From Array(array=w1023, length=1 ("长度"), index (col)=3 ("禁用的索引 (列)")) -> (array with subset deleted=w1020:string[][])  [unwired: 1 in, 1 out]
          n480 = Insert Into Array(array=w1020, index (col)=3 ("禁用的索引 (列)"), new element=w1019) -> (w1017:string[][])  [unwired: 1 in]
        }
      }
    }
  }
  "待发送数据" <- w1
  "columns输出" <- w2
  n481 = call <vilib>:"Clear Errors.vi"("error in (no error)"=w8) -> ("error out"=→"error out":errorcluster)  [unwired: 5 in, 1 out]
  n482 = Index Array(array=w1, index (row)=0 ("索引 (行)")) -> (element=→"待发送第一条数据":string[])  [unwired: 1 in]
